vi "GIS Head Poll Process.vi"(7 "HeadNo":string, 8 "error in (no error)":errorcluster, 9 "notifierSync":refnum<notifier>, 10 "TopLevel":refnum<class "TopLevel.lvclass">, 11 "GIS Printer in":refnum<class "GIS Printer.lvclass">) -> (0 "error out":errorcluster, 3 "GIS Printer out":refnum<class "GIS Printer.lvclass">)   [LabVIEW 2022 SP3, in "GIS Printer.lvclass"]
uses:
  GIS Printer.lvclass
  TopLevel/TopLevel.lvclass
  Typedefs/PollCommandData-Cluster.ctl
  Typedefs/GIS_PollTimers--cluster.ctl
panel:
  in  "C1":bool
  in  "A1":bool
  in  "C2":bool
  in  "A2":bool
  in  "C3":bool
  in  "A3":bool
  in  "C4":bool
  in  "A4":bool
  in  "C33":bool
  in  "I33 3":bool
  in  "I33 2":bool
  in  "I33 1":bool
  in  "A33":bool
  in  "C22":bool
  in  "A22":bool
  in  "C11":bool
  in  "A11":bool
  in  "OK":bool
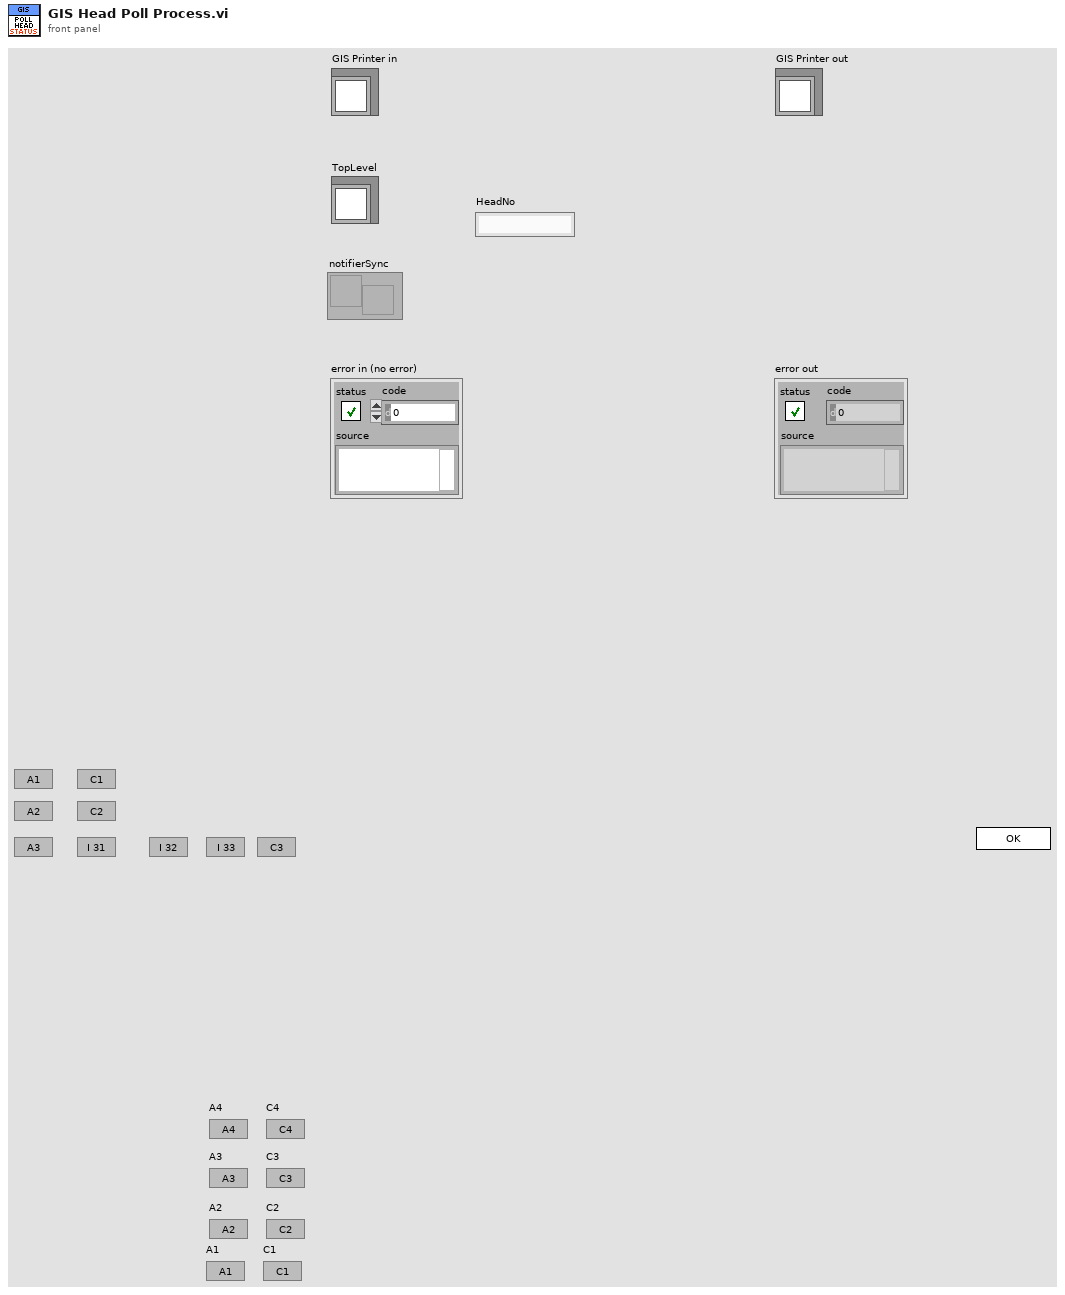
[diagram p1: front panel]
types:
  T1 = typedef "PollCommandData-Cluster.ctl" = cluster{"Command":string, "ID":i32, "Complete":bool}
  T2 = cluster{"String":string, "PrinterPollResponse":refnum<user-event>, "Open":bool, "TCP":refnum<k5>, "PollTrk":cluster{"CurrentCmdIndex":i32, "TotalCommands":i32}, "PollCommands":string[]}
  T3 = typedef "TD Dynamic CVT DVR--ref.ctl" = refnum<data-value>
  T4 = enum32{"Invalid", "Standard", "Closed", "Hidden", "Minimized", "Maximized"}
  T5 = enum32{"invalid app kind", "Development System", "Run Time System", "Student Edition", "Embedded LabVIEW", "Evaluation", "Custom"}
  T6 = typedef "GIS Printer.lvclass/PrinterConfiguration--Cluster.ctl" = cluster{"IPAddress":string, "Move Stage on RTP Command?":bool, "Stage Move Position":string, "PH1-Prime Path":path, "PH2-Prime Path":path, "PH3-Prime Path":path, "PH4-Prime Path":path, "PH5-Prime Path":path, "PH6-Prime Path":path, "PrintScriptsFolder":path, "PurgeScriptsFolder":path, "StageScriptsFolder":path, "PH1-HeatOn Path":path, "PH2-HeatOn Path":path, "PH3-HeatOn Path":path, "PH4-HeatOn Path":path, "PH5-HeatOn Path":path, "PH6-HeatOn Path":path, "PH1-HeatOff Path":path, "PH2-HeatOff Path":path, "PH3-HeatOff Path":path, "PH4-HeatOff Path":path, "PH5-HeatOff Path":path, "PH6-HeatOff Path":path}
  T7 = typedef "GIS_PollTimers--cluster.ctl" = cluster{"HeadStatus":dbl}
  T8 = cluster{"GIS Printer in":refnum<class "GIS Printer.lvclass">, "Core":cluster{"Current VI Reference":refnum<vi>, "Close Panel on Exit?":bool}, "PrinterConfiguration":T6, "TCP":refnum<k5>, "PollTimers":T7, "PollTracker":cluster{"HeadStatusPollStart":dbl, "Poll":bool}, "notifierSync":refnum<notifier>, "PollEnable":bool}
  T9 = cluster{"Current VI Reference":refnum<vi>, "Close Panel on Exit?":bool}
  T10 = typedef "TopLevel.lvclass/Digilens Config Cluster.ctl" = cluster{"Motion Controller":T11, "IO Config":T12, "PrinterConfiguration":T6, "DAQ Settings":T15}
  T11 = typedef "Motor Controller.lvclass/Motor Controller Config Data.ctl" = cluster{"Motor IP Addresss":string, "Current Position":i32, "Pulse_Per_mm":i32, "PrePrint":dbl[], "Load Position_mm":i32, "Laminate Position_mm":i32}
  T12 = typedef "IO.lvclass/IO Config Data.ctl" = cluster{"DAQDevices":T13[], "DI Channels":T14[], "DO Channels":T14[], "Material Names":string[], "AI Channels":T14[], "AO Channels":T14[]}
  T13 = typedef "IO.lvclass/DCON_DeviceConfig--Cluster.ctl" = cluster{"COM":string, "DeviceName":string, "BaudRate":u32, "Number of Channels":i32, "DeviceAddress":i32, "Enable":bool}
  T14 = typedef "IO.lvclass/Channel Data.ctl" = cluster{"Channel Name":string, "Device Name":string, "Channel No":string}
  T15 = typedef "DAQ.lvclass/TD DAQ Settings--cluster.ctl" = cluster{"Simulate DAQ":bool, "DI Settings":T16[], "AI Settings":T17[], "Relay IONames":string[], "AO IONames":string[], "AO NChan SingleTask":bool}
  T16 = typedef "DAQ.lvclass/TD DI Instrument Settings--cluster.ctl" = cluster{"Disable":bool, "DI TaskName":string, "DI RefreshIntv":i32}
  T17 = typedef "DAQ.lvclass/TD AI Instrument Settings--cluster.ctl" = cluster{"Disable":bool, "AI TaskName":string, "AI InstSettings":T18, "SimAI Ranges":T19}
  T18 = typedef "DAQ.lvclass/TD AI InstSettings--cluster.ctl" = cluster{"DaqRate":dbl, "NumSamples":i32}
  T19 = typedef "DAQ.lvclass/TD SimAI Ranges--cluster.ctl" = cluster{"lo":dbl, "hi":dbl}
  T20 = typedef "TopLevel.lvclass/UserEvents.ctl" = cluster{"API Incoming Event":refnum<user-event>, "API Executed Event":refnum<user-event>, "API Return Event":refnum<user-event>, "Exit Event":refnum<user-event>, "StatusChanged":refnum<user-event>, "DLP GUI Config Changed":refnum<user-event>, "AppEvent":refnum<user-event>, "Login Event":refnum<user-event>}
  T21 = typedef "GIS Printer.lvclass/UserEvents.ctl" = cluster{"API Incoming Event":refnum<user-event>, "API Executed Event":refnum<user-event>, "API Return Event":refnum<user-event>, "Status Changed Event":refnum<user-event>, "Abort":refnum<user-event>, "stop process":refnum<user-event>, "GISPollStatus":refnum<user-event>, "GISHeadStatus":refnum<user-event>, "Error Event":refnum<user-event>}
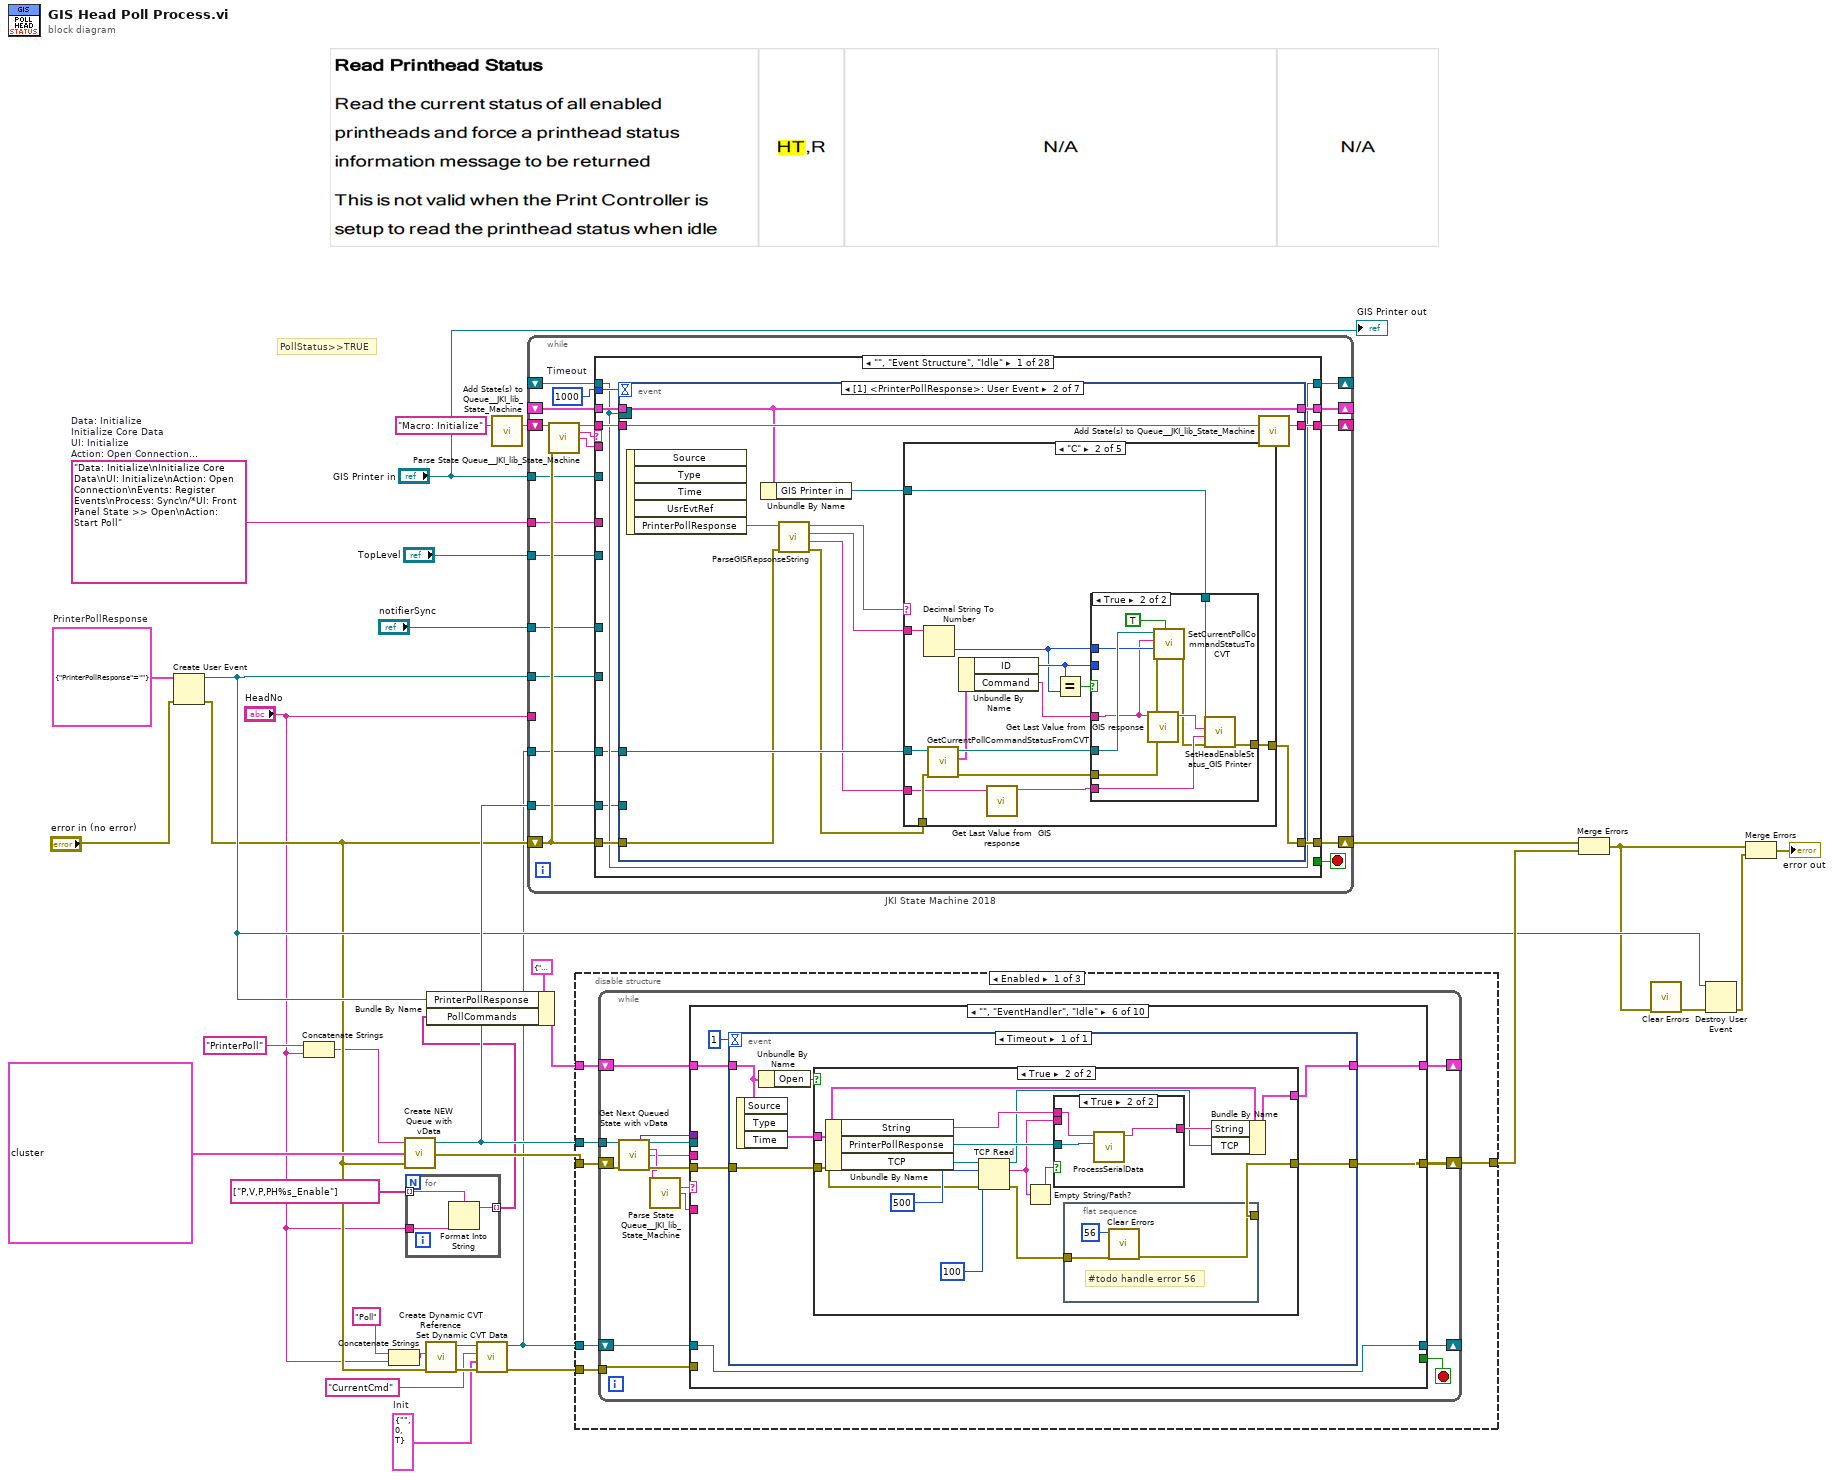
[diagram p0: block diagram]
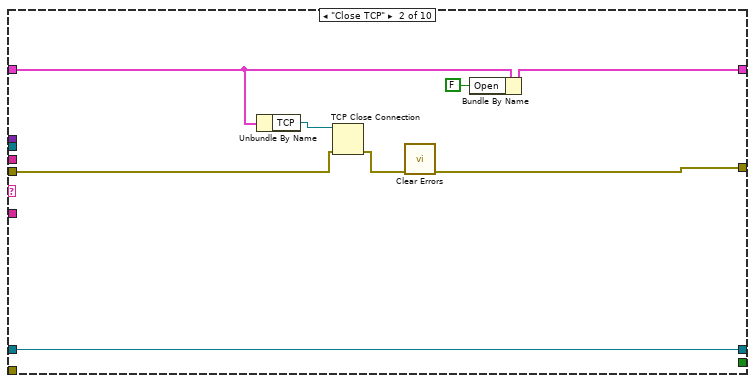
[diagram p3: hidden frame]
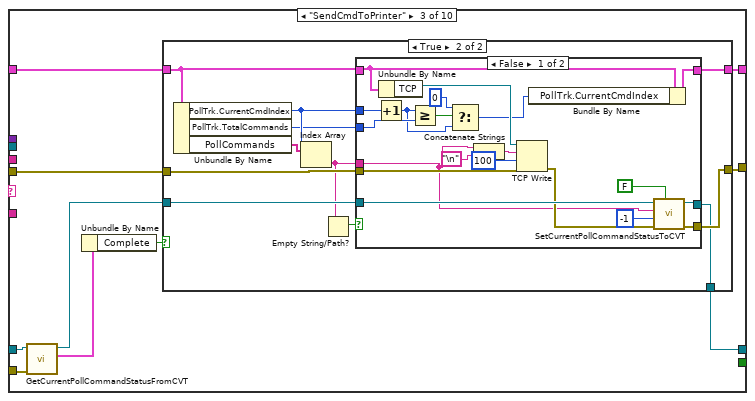
[diagram p4: hidden frame]
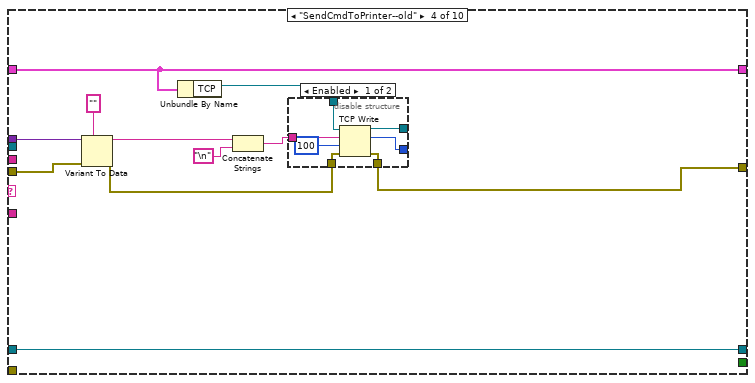
[diagram p7: hidden frame]
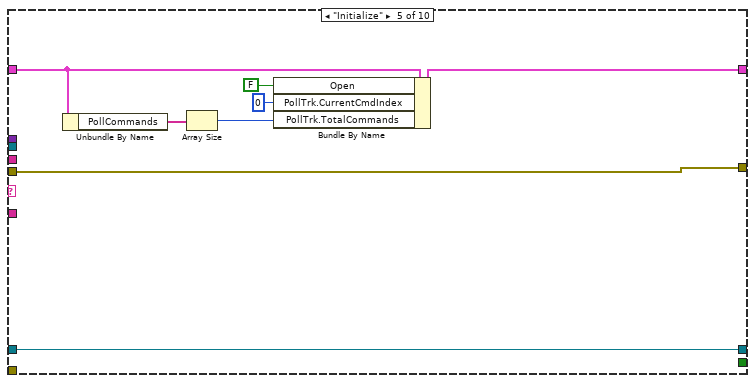
[diagram p9: hidden frame]
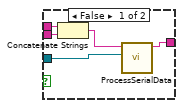
[diagram p11: hidden frame]
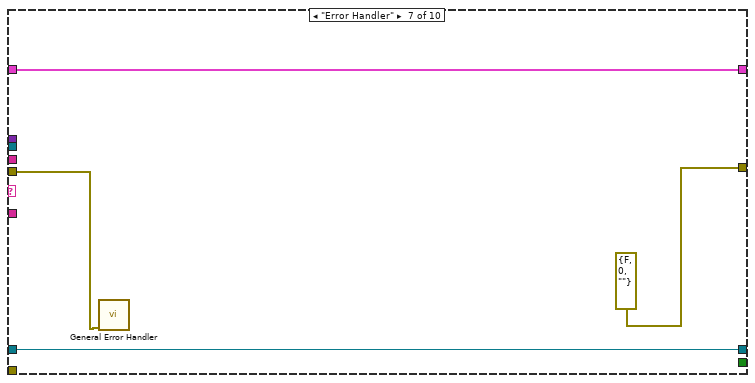
[diagram p12: hidden frame]
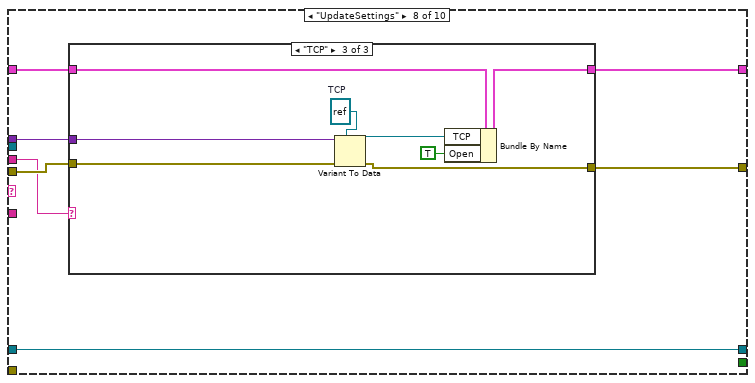
[diagram p13: hidden frame]
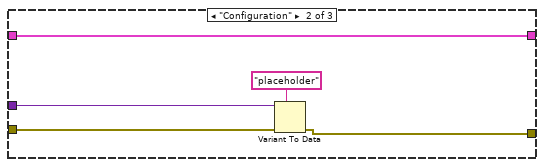
[diagram p15: hidden frame]
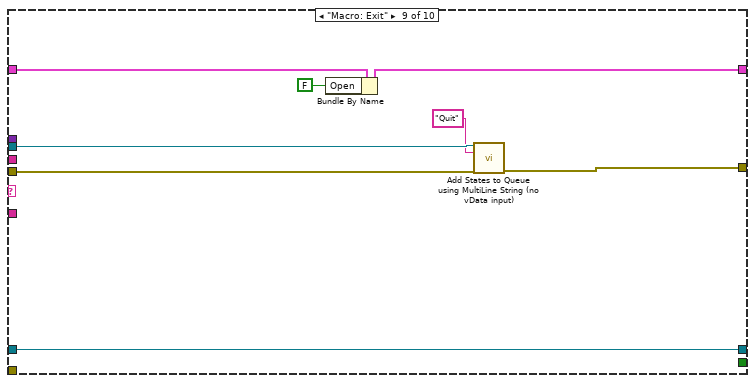
[diagram p16: hidden frame]
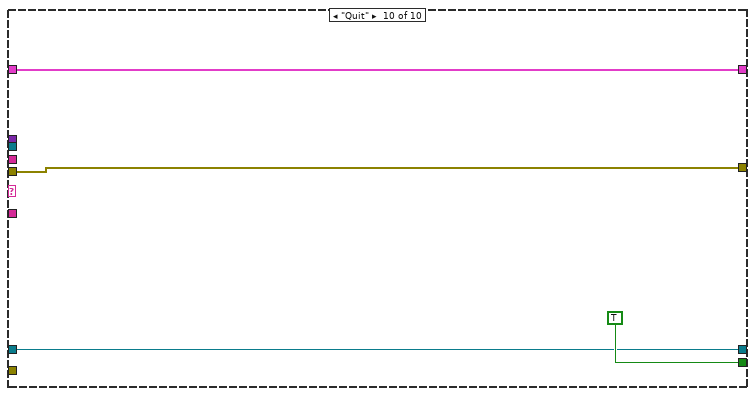
[diagram p17: hidden frame]
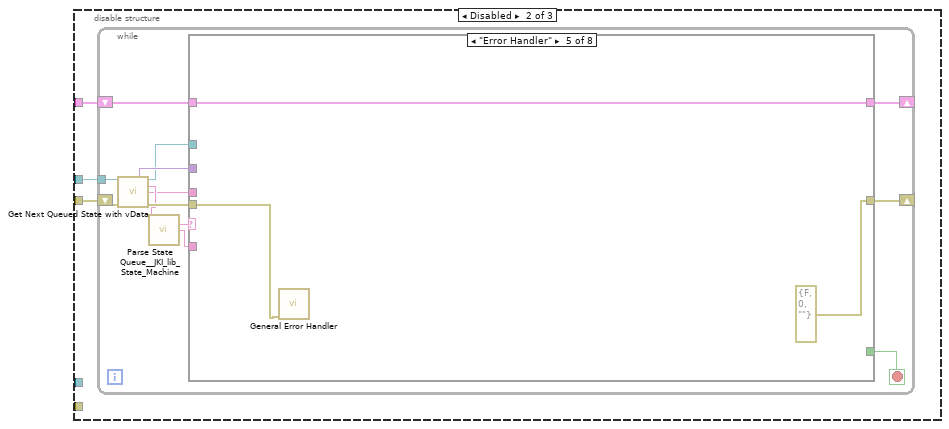
[diagram p18: hidden frame]
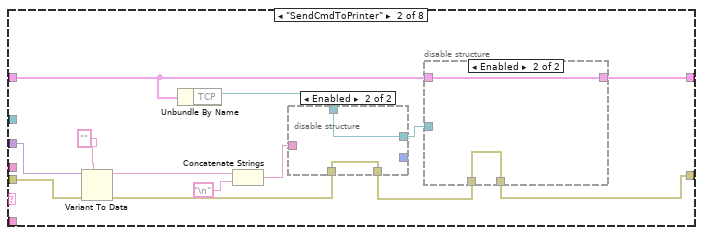
[diagram p20: hidden frame]
diagram:
  w7 = T1 {"Command"="", "ID"=0, "Complete"=TRUE}  # Init
  w14 = "Data: Initialize\nInitialize Core Data\nUI: Initialize\nAction: Open Connection\nEvents: Register Events\nProcess: Sync\n/*UI: Front Panel State >> Open\nAction: Start Poll"  # Data: Initialize Initialize Core Data UI: Initialize Action: Open Connection Events: Register Events Process: Sync /*UI: Front Panel State >> Open Action: Start Poll
  w25 = cluster{"PrinterPollResponse":string} {"PrinterPollResponse"=""}  # PrinterPollResponse
  # "PollStatus>>TRUE"
  n1 = Create User Event(user event datatype=w25, error in="error in (no error)") -> (user event=w22:refnum<user-event>, error out=w8:errorcluster)
  n2 = Concatenate Strings("PrinterPoll" ("Name (SMQ)"), "HeadNo") -> (w5:string)
  n3 = Concatenate Strings("Poll" ("DictName"), "HeadNo") -> (w4:string)
  n4 = call <vilib>:"Create NEW Queue with vData.vi"("error in (no error)"=w8, "Initial States"=cluster{"state":string, "vData":variant}[] [{"state"="Initialize", "vData"=variant}, {"state"="Idle", "vData"=variant}], "Name (SMQ)"=w5) -> ("error out"=w30:errorcluster, "queue out"=w26:refnum<queue>)  [unwired: 1 in]
  n5 = for {
    tunnel: string[] ["P,V,P,PH%s_Enable"] -> [w37] mode=indexing
    tunnel: "HeadNo" -> [w36]
    tunnel: [w35] -> w1 mode=indexing
    n6 = Format Into String(format string=w37, w36) -> (resulting string=w35:string)  [unwired: 2 in, 1 out]
  }
  n7 = call <vilib>:"Create Dynamic CVT Reference.vi"("error in (no error)"=w8, "DictName"=w4) -> ("error out"=w11:errorcluster, "dCVT DVR out"=w12:T3)  [unwired: 8 in]
  n8 = Bundle By Name(cluster=T2 {"String"="", "PrinterPollResponse"=refnum, "Open"=FALSE, "TCP"=refnum, "PollTrk"={"CurrentCmdIndex"=0, "TotalCommands"=0}, "PollCommands"=[]}, "PrinterPollResponse"=w22, "PollCommands"=w1) -> (w27:T2)
  n9 = call <vilib>:"Set Dynamic CVT Data.vi"("error in (no error)"=w11, "value"=w7, "DataName"="CurrentCmd", "dCVT DVR"=w12) -> ("error out"=w10:errorcluster, "dCVT DVR out"=w6:T3)  [unwired: 5 in, 1 out]
  n10 = call <vilib>:"Add State(s) to Queue__JKI_lib_State_Machine.vi"("State(s) in (\"\")"="Macro: Initialize") -> ("States Out"=w34:string)  [unwired: 14 in]
  n11 = while "JKI State Machine 2018" {
    shift-right: [w50] -> _
    shift-left: _ -> [w49]
    shift-right: [w53] -> w24
    shift-left: w8 -> [w47]
    shift-right: [w52] -> _
    shift-left: w34 -> [w54]
    tunnel: "GIS Printer in" -> [w46]
    tunnel: "TopLevel" -> [w45]
    tunnel: w26 -> [w44]
    tunnel: w22 -> [w43]
    shift-right: [w42] -> _
    shift-left: _ -> [w41]
    tunnel: "notifierSync" -> [w40]
    tunnel: w14 -> [w39]
    tunnel: w6 -> [w38]
    tunnel: "HeadNo" -> [_]
    stop <- w51 stop-if-true
    w48 = 1000  # Timeout
    n12 = call <vilib>:"Parse State Queue__JKI_lib_State_Machine.vi"("State Queue"=w54, "Error In (no error)"=w47) -> ("Remaining States"=w56:string, "Current State"=w57:string, "Arguments"=w55:string)  [unwired: 11 in]
    n13 = case shown="\"\", \"Event Structure\", \"Idle\"" w57 {
      selector: w57 -> [_ _ w182 _ _ _ _ _ _ _ _ _ _ _ _ _ _ _ _ _ _ _ _ _ _ _ _ _]
      tunnel: w56 -> [w67 w180 w186 w206 w213 w222 w227 w234 w248 w263 w270 w275 w280 w287 w299 w369 w375 w386 w391 w399 w407 w421 w435 w444 w459 w465 w477 w488]
      tunnel: w55 -> [_ _ _ _ _ _ _ _ _ _ _ _ _ w282 w293 _ _ _ _ _ _ _ _ _ _ _ w473 _]
      tunnel: w49 -> [w65 w177 w184 w199 w210 w220 w224 w232 w241 _ w265 w272 w278 w285 w295 w366 w372 w383 w388 w396 w402 w417 w431 w441 w454 w463 w475 w478]
      tunnel: [w64 w178 w188 w203 errorcluster {"status"=FALSE, "code"=0, "source"=""} ("error out") w215 w225 w230 w237 w249 w266 w273 w277 w283 w296 w367 w373 w384 w389 w393 w401 w419 w433 w442 w450 w461 w471 w481] -> w53
      tunnel: w47 -> [w63 w178 w187 w203 w209 w214 w225 w229 w243 w249 w267 w273 w277 w284 w297 w367 w373 w384 w389 w392 w400 w419 w433 w442 w446 w460 w470 w480]
      tunnel: [w66 w179 w185 w205 w212 w221 w226 w233 w247 w262 w269 w274 w279 w286 w298 w368 w374 w385 w390 w398 w406 w420 w434 w443 w458 w464 w476 w487] -> w52
      tunnel: [_ _ _ _ _ TRUE _ _ _ _ _ _ _ _ _ _ _ _ _ _ _ _ _ _ _ _ _ _] -> w51
      tunnel: [w62 w177 w184 w204 w210 w220 w224 w232 w242 w261 w265 w272 w278 w285 w295 w366 w372 w383 w388 w396 w402 w417 w431 w439 w454 w463 w468 w479] -> w50
      tunnel: w48 -> [w61 _ _ _ _ _ _ _ _ _ _ _ _ _ _ _ _ _ _ _ _ _ _ _ _ _ _ _]
      tunnel: w46 -> [_ _ _ _ _ _ _ _ _ w250 _ _ _ _ _ _ _ _ _ _ _ _ _ _ _ _ _ _]
      tunnel: w45 -> [_ _ _ _ _ _ _ _ _ w259 _ _ _ _ _ _ _ _ _ _ _ _ _ _ w448 _ _ _]
      tunnel: w44 -> [w58 _ _ _ _ w216 _ _ w239 _ _ _ _ _ _ _ _ _ _ w394 _ _ _ _ _ _ w472 w482]
      tunnel: w43 -> [_ _ _ _ _ _ _ _ _ _ _ _ _ _ _ _ _ _ _ _ _ _ _ _ w457 _ _ _]
      tunnel: [w60 w176 w181 w193 w207 w218 w223 w228 w235 w255 w264 w271 w276 w281 w292 w365 w371 w376 w387 w397 w405 w418 w432 w440 w456 w462 w469 w486] -> w42
      tunnel: w41 -> [w60 w176 w181 w193 w207 w218 w223 w228 w235 w255 w264 w271 w276 w281 w292 w365 w371 w376 w387 w397 w405 w418 w432 w440 _ w462 w469 w486]
      tunnel: w40 -> [_ _ _ _ _ _ _ _ _ w252 _ _ _ _ _ _ _ _ _ _ _ _ _ _ _ _ _ _]
      tunnel: w39 -> [_ _ _ _ _ _ _ _ _ _ _ _ _ _ _ _ w370 _ _ _ _ _ _ _ _ _ _ _]
      tunnel: w38 -> [w59 _ _ _ _ _ _ _ _ _ _ _ _ _ _ _ _ _ _ _ _ _ _ _ _ _ _ _]
      frame "", "Event Structure", "Idle" {
        n14 = event shown="[1] <PrinterPollResponse>: User Event" {
          selector: w60 -> [_ _ _ _ _ _ _]
          dyn-events: _ -> [_ _ _ _ _ _ _]
          timeout: w61 -> [_ _ _ _ _ _ _]
          tunnel: w67 -> [w75 w88 w143 w148 w152 w160 w175]
          tunnel: [w74 w87 w142 w147 w151 w159 w174] -> w66
          tunnel: w65 -> [w71 w84 w140 w145 w149 w155 w172]
          tunnel: [w73 w82 w141 w146 w150 w154 w173] -> w64
          tunnel: w63 -> [w73 w77 w141 w146 w150 w153 w173]
          tunnel: [w71 w84 w140 w145 w149 w156 w172] -> w62
          tunnel: w59 -> [_ w81 _ _ _ _ _]
          tunnel: w58 -> [_ _ _ _ _ _ _]
          event Timeout {
            n15 = event-data() -> ()  [unwired: 1 in, 1 out]
            n16 = Unbundle By Name(w71) -> ("PollTracker.Poll"=w70:bool, "PollEnable"=w68:bool)
            n17 = And(x=w70, y=w68) -> (x .and. y?=w69:bool)
            n18 = case shown="True" w69 {
              tunnel: [_ "Action: CheckPollTimers" ("State(s) in Front (\"\")")] -> w72
              frame False {
              }
              frame True {
              }
            }
            n19 = call <vilib>:"Add State(s) to Queue__JKI_lib_State_Machine.vi"("State(s) in Front (\"\")"=w72, "State(s) in (\"\")"=w75) -> ("States Out"=w74:string)  [unwired: 13 in]
          }
          event User Event {
            n20 = event-data() -> ("PrinterPollResponse"=w86:string)  [unwired: 1 in, 4 out]
            n21 = Unbundle By Name(w84) -> ("GIS Printer in"=w83:refnum<class "GIS Printer.lvclass">)
            n22 = call "ParseGISRepsonseString.vi"("error in (no error)"=w77, "Response In"=w86) -> ("error out"=w78:errorcluster, "Status"=w79:string, "ID"=w80:string, "Category"=w85:string)  [unwired: 6 in]
            n23 = case shown="\"C\"" w85 {
              tunnel: w79 -> [_ w91 w118 _ _]
              tunnel: w83 -> [_ w94 _ w137 _]
              tunnel: w78 -> [w89 w96 w124 w133 w138]
              tunnel: [w89 w97 w121 w134 w138] -> w82
              tunnel: w81 -> [_ w98 w125 _ _]
              tunnel: w80 -> [_ w92 w119 _ _]
              frame Default {
              }
              frame "C" {
                n24 = Decimal String To Number(string=w92) -> (number=w99:i32)  [unwired: 2 in, 1 out]
                n25 = call "GetCurrentPollCommandStatusFromCVT.vi"("error in (no error)"=w96, "Data Value Reference in"=w98) -> ("error out"=w102:errorcluster, "Command"=w95:T1, "Data Value Reference out"=w103:T3)  [unwired: 7 in]
                n26 = Unbundle By Name(w95) -> ("ID"=w100:i32, "Command"=w93:string)
                n27 = call "Get Last Value from  GIS response.vi"("Command"=w91) -> ("String"=w90:string)  [unwired: 10 in]
                n28 = Equal?(x=w100, y=w99) -> (x = y?=w101:bool)
                n29 = case shown="True" w101 {
                  tunnel: w103 -> [_ w114]
                  tunnel: w102 -> [w104 w113]
                  tunnel: [w104 w105] -> w97
                  tunnel: w100 -> [_ _]
                  tunnel: w99 -> [_ w111]
                  tunnel: w93 -> [_ w109]
                  tunnel: w94 -> [_ w110]
                  tunnel: w90 -> [_ w107]
                  frame False {
                    # "Ack is for a\ndifferent cmd,\nshould never\nhappen"
                  }
                  frame True {
                    n30 = call "Get Last Value from  GIS response.vi"("Command"=w109) -> ("String"=w108:string)  [unwired: 10 in]
                    n31 = call "SetCurrentPollCommandStatusToCVT.vi"("Complete"=TRUE, "error in (no error)"=w113, "Ack"=w111, "Command"=w109, "Data Value Reference in"=w114) -> ("error out"=w106:errorcluster)  [unwired: 5 in, 1 out]
                    n32 = call-dynamic "SetHeadEnableStatus_GIS Printer.vi"("error in (no error)"=w106, "Value"=w107, "Command"=w108, "GIS Printer In"=w110) -> ("error out"=w105:errorcluster)  [unwired: 6 in, 1 out]
                  }
                }
              }
              frame "A" {
                n33 = Decimal String To Number(string=w119) -> (number=w115:i32)  [unwired: 2 in, 1 out]
                n34 = call "GetCurrentPollCommandStatusFromCVT.vi"("error in (no error)"=w124, "Data Value Reference in"=w125) -> ("error out"=w122:errorcluster, "Command"=w120:T1, "Data Value Reference out"=w123:T3)  [unwired: 7 in]
                n35 = Unbundle By Name(w120) -> ("Command"=w116:string)
                n36 = Equal?(x=w116, y=w118) -> (x = y?=w117:bool)
                n37 = case shown="False" w117 {
                  tunnel: w123 -> [_ w132]
                  tunnel: w122 -> [w126 w131]
                  tunnel: [w126 w130] -> w121
                  tunnel: w120 -> [_ _]
                  tunnel: w116 -> [_ w128]
                  tunnel: w115 -> [_ w127]
                  frame False {
                    # "Ack is for a\ndifferent cmd,\nshould never\nhappen"
                  }
                  frame True {
                    n38 = call "SetCurrentPollCommandStatusToCVT.vi"("Complete"=FALSE, "error in (no error)"=w131, "Ack"=w127, "Command"=w128, "Data Value Reference in"=w132) -> ("error out"=w130:errorcluster)  [unwired: 5 in, 1 out]
                  }
                }
              }
              frame "E" {
                # "Should be replaced with actual error"
                n39 = call-dynamic "Generate Error Event.vi"("Error"=errorcluster {"status"=FALSE, "code"=0, "source"=""}, "GIS Printer in"=w137) -> ("error out"=w136:errorcluster)  [unwired: 8 in, 1 out]
                n40 = Merge Errors(w133, w136) -> (w134:errorcluster)
              }
              frame "I" {
              }
            }
            n41 = call <vilib>:"Add State(s) to Queue__JKI_lib_State_Machine.vi"("State(s) in (\"\")"=w88) -> ("States Out"=w87:string)  [unwired: 14 in]
          }
          event "OK": Value Change {
            # "Exit Button Value Change (pressed) Event\n(this executes Macro: Exit to terminate the VI)"
            n42 = event-data() -> ()  [unwired: 1 in, 1 out]
            n43 = call <vilib>:"Add State(s) to Queue__JKI_lib_State_Machine.vi"("State(s) in Front (\"\")"="Macro: Exit", "State(s) in (\"\")"=w143) -> ("States Out"=w142:string)  [unwired: 13 in]
          }
          event User Event {
            # "Exit Button Value Change (pressed) Event\n(this executes Macro: Exit to terminate the VI)"
            n44 = event-data() -> ()  [unwired: 1 in, 5 out]
            n45 = call <vilib>:"Add State(s) to Queue__JKI_lib_State_Machine.vi"("State(s) in Front (\"\")"="Macro: Exit", "State(s) in (\"\")"=w148) -> ("States Out"=w147:string)  [unwired: 13 in]
          }
          event User Event {
            # "#TODO API: Abort called in  other process. do something about it man!\njust do something...anything"
            # "Exit Button Value Change (pressed) Event\n(this executes Macro: Exit to terminate the VI)"
            n46 = event-data() -> ()  [unwired: 1 in, 5 out]
            n47 = call <vilib>:"Add State(s) to Queue__JKI_lib_State_Machine.vi"("State(s) in (\"\")"=w152) -> ("States Out"=w151:string)  [unwired: 14 in]
          }
          event User Event {
            n48 = event-data() -> ("Command"=w158:string, "Data"=w157:variant)  [unwired: 1 in, 4 out]
            n49 = case shown="\"StatusPoll\"" w158 {
              tunnel: w157 -> [_ w169]
              tunnel: w155 -> [w162 w167]
              tunnel: [w162 w166] -> w156
              tunnel: w153 -> [w161 w164]
              tunnel: [w161 w163] -> w154
              frame Default {
              }
              frame "StatusPoll" {
                n50 = Variant To Data(error in=w164, type=FALSE, Variant=w169) -> (data=w165:bool, error out=w163:errorcluster)
                n51 = Bundle By Name(cluster=w167, "PollEnable"=w165) -> (w166:T8)
              }
            }
            n52 = call <vilib>:"Add State(s) to Queue__JKI_lib_State_Machine.vi"("State(s) in (\"\")"=w160) -> ("States Out"=w159:string)  [unwired: 14 in]
          }
          event Panel Close? {
            # "Discard the event because we'll close the front panel ourselves in Macro: Exit"
            # "Close Panel button (pressed) Event\n(this executes Macro: Exit to terminate the VI)"
            n53 = event-data() -> ()  [unwired: 1 in, 1 out]
            n54 = event-data("Discard?"=TRUE) -> ()  [unwired: 1 in, 1 out]
            n55 = call <vilib>:"Add State(s) to Queue__JKI_lib_State_Machine.vi"("State(s) in Front (\"\")"="Macro: Exit", "State(s) in (\"\")"=w175) -> ("States Out"=w174:string)  [unwired: 13 in]
          }
        }
      }
      frame "---------- Core ----------" {
        # "Do not put any code in this frame.\n(it is a separator no-op)"
        n56 = call <vilib>:"Add State(s) to Queue__JKI_lib_State_Machine.vi"("State(s) in (\"\")"=w180) -> ("States Out"=w179:string)  [unwired: 14 in]
      }
      frame Default {
        w191 = 42 items=["No error", "Argument error", "Memory is full", "Out of zone", "End of file", "File already open", "Generic file I/O error", "File not found", "File permission error", "Disk is full", "Duplicate path", "Too many files open", "System feature not enabled", "Resource file not found", "Cannot add resource", "Resource not found", "Image not found", "Image memory error", "Pen does not exist", "Config type invalid", "Config token not found", "Config parse error", "Config memory error", "Bad external code format", "Bad external code offset", "External code not present", "Null window", "Destroy window error", "Null menu", "Print aborted", "Bad print record", "Print driver error", "Windows error during printing", "Memory error during printing", "Print dialog error", "Generic print error", "Invalid device refnum", "Device not found", "Device parameter error", "Device unit error", "Cannot open device", "Device call aborted", "Generic error", "Cancelled by user", "Object ID too low", "Object ID too high", "Object not in heap", "Unknown heap", "Unknown object (invalid DefProc)", "Unknown object (DefProc not in table)", "Message out of range", "Invalid (null) method", "Unknown message", "Manager call not supported", "Bad address", "Network operation in progress", "Network operation timed out", "Connection is busy", "Network attribute not supported", "Network error", "Address in use", "System out of memory", "Connection aborted", "Connection refused", "Not connected", "Already connected", "Connection closed", "Initialization error (interapplication manager)", "Bad occurrence", "Wait on unbound occurrence handler", "Occurrence queue overflow", "Datalog type conflict", "Unused", "Unrecognized type (interapplication manager)", "Memory corrupt", "Failed to make temporary DLL", "Old CIN version", "Drag socket not found", "Failed to load drop-object", "Failed to register OLE object", "Failed to release OLE object", "Format specifier type mismatch", "Unknown format specifier", "Too few format specifiers", "Too many format specifiers", "Scan failed", "Newer CIN version", "Error converting to variant", "Runtime menu error", "Password tampered", "Variant attribute not found", "Incompatible variant data type", "Event data is not available", "Event Store is not present", "Occurrence is not found", "Event Queue is not created", "Event info is not available", "Refnum passed is NULL", "Error retrieving Class GUID", "Error retrieving CoClass GUID", "Error retrieving TypeLib GUID.", "Bad built application magic bytes.", "Specific driver is different from the specific driver associated with the Logical Name.", "There is no session opened to the class driver.", "Max Error", "MAX - Error with config objects", "MAX - Error loading configuration", "MAX - Group not supported"]
        # "Current State"
        # "Do not delete, rename, or modify this frame.\n(this is used to capture unhandled states and typos)"
        # "Handle mistyped state name (developer tool)"
        n57 = Format Into String(format string="Software Exception: Unhandled State \"%s\"." ("message"), error in=w187, w182) -> (resulting string=w190:string, error out=w189:errorcluster)  [unwired: 1 in]
        n58 = call <vilib>:"Error Cluster From Error Code.vi"("show call chain? (False)"=TRUE, "error in (no error)"=w189, "error message (\"\")"=w190, "error code (0)"=w191) -> ("error out"=w188:errorcluster)  [unwired: 5 in]
        n59 = call <vilib>:"Add State(s) to Queue__JKI_lib_State_Machine.vi"("State(s) in (\"\")"=w186) -> ("States Out"=w185:string)  [unwired: 14 in]
      }
      frame "Initialize Core Data" {
        # "Do not delete, rename, or modify this frame.\n(this is used to determine panel behavior on exit)"
        # "originally closed?"
        # "exe?"
        # "If panel starts closed or is an EXE, then close it when we exit"
        n60 = property class="VI"() -> ("FP.State"=w196:T4)  [unwired: 2 in, 2 out]
        n61 = property class="App"() -> ("App.Kind"=w202:T5)  [unwired: 2 in, 2 out]
        n62 = control-ref of="Current VI Reference"() -> (w197:refnum<vi>)
        n63 = Equal?(x=w196, y=T4."Closed" ("Front Panel Window:State")) -> (x = y?=w194:bool)
        n64 = Equal?(x=w202, y=T5."Run Time System" ("Application:Kind")) -> (x = y?=w200:bool)
        n65 = Or(x=w194, y=w200) -> (x .or. y?=w198:bool)
        n66 = Bundle By Name(cluster=w199, "Core.Current VI Reference"=w197, "Core.Close Panel on Exit?"=w198) -> (w204:T8)
        n67 = call <vilib>:"Add State(s) to Queue__JKI_lib_State_Machine.vi"("State(s) in (\"\")"=w206) -> ("States Out"=w205:string)  [unwired: 14 in]
      }
      frame "Error Handler" {
        # "Unhandled Error -- Display it"
        # "Handle any errors here.\nYou can also output any states to clean-up after errors occur"
        # "Clear error"
        n68 = call <vilib>:"General Error Handler.vi"("error in (no error)"=w209) -> ()  [unwired: 10 in, 5 out]
        n69 = call <vilib>:"Add State(s) to Queue__JKI_lib_State_Machine.vi"("State(s) in Front (\"\")"="/* Post Error States", "State(s) in (\"\")"=w213) -> ("States Out"=w212:string)  [unwired: 13 in]
      }
      frame "Exit" {
        n70 = call <vilib>:"Add States to Queue using MultiLine String (no vData input).vi"("queue in"=w216, "states in"="Quit", "error in"=w214) -> ("error out"=w215:errorcluster)  [unwired: 10 in, 2 out]
        n71 = call <vilib>:"Add State(s) to Queue__JKI_lib_State_Machine.vi"("State(s) in (\"\")"=w222) -> ("States Out"=w221:string)  [unwired: 14 in]
      }
      frame "---------- Data ----------" {
        # "Do not put any code in this frame.\n(It is a separator no-op. You can make a copy of this frame to create a new Data frame)"
        n72 = call <vilib>:"Add State(s) to Queue__JKI_lib_State_Machine.vi"("State(s) in (\"\")"=w227) -> ("States Out"=w226:string)  [unwired: 14 in]
      }
      frame "Data: GIS Disconnect" {
        # "Do not put any code in this frame.\n(It is a separator no-op. You can make a copy of this frame to create a new Data frame)"
        n73 = Unbundle By Name(w232) -> ("TCP"=w231:refnum<k5>)
        n74 = TCP Close Connection(connection ID=w231, error in (no error)=w229) -> (error out=w230:errorcluster)  [unwired: 1 in, 1 out]
        n75 = call <vilib>:"Add State(s) to Queue__JKI_lib_State_Machine.vi"("State(s) in (\"\")"=w234) -> ("States Out"=w233:string)  [unwired: 14 in]
      }
      frame "Data: GIS Connect" {
        n76 = Unbundle By Name(w241) -> ("PrinterConfiguration.IPAddress"=w246:string)
        n77 = TCP Open Connection(address=w246, remote port or service name=u16 2000, timeout ms (60000)=1000, error in (no error)=w243) -> (connection ID=w236:refnum<k5>, error out=w238:errorcluster)  [unwired: 1 in]
        n78 = call <vilib>:"Add State to Queue with vData.vi"("queue in"=w239, "state in"="UpdateSettings>>TCP", "vData (\"\")"=w236, "error in"=w238) -> ("error out"=w237:errorcluster)  [unwired: 8 in, 3 out]
        n79 = Bundle By Name(cluster=w241, "TCP"=w236) -> (w242:T8)
        n80 = call <vilib>:"Add State(s) to Queue__JKI_lib_State_Machine.vi"("State(s) in (\"\")"=w248) -> ("States Out"=w247:string)  [unwired: 14 in]
      }
      frame "Data: Initialize" {
        w251 = TRUE  # PollEnable
        w253 = cluster{"HeadStatusPollStart":dbl, "Poll":bool} {"HeadStatusPollStart"=0.0, "Poll"=FALSE}  # PollTracker
        w254 = T7 {"HeadStatus"=2.0}  # PollTimers
        w256 = refnum<k5> refnum  # TCP
        w260 = T9 {"Current VI Reference"=refnum, "Close Panel on Exit?"=FALSE}  # Core
        # "#TODO get from config"
        n81 = property class="TopLevel.lvclass"(reference=w259) -> ("Methods:Accessors:Digilens Config"=w258:T10)  [unwired: 1 in, 2 out]
        n82 = Unbundle By Name(w258) -> ("PrinterConfiguration"=w257:T6)
        n83 = Bundle("GIS Printer in"=w250, "Core"=w260, "PrinterConfiguration"=w257, "TCP"=w256, "PollTimers"=w254, "PollTracker"=w253, "notifierSync"=w252, "PollEnable"=w251) -> (w261:T8)  [unwired: 1 in]
        n84 = call <vilib>:"Add State(s) to Queue__JKI_lib_State_Machine.vi"("State(s) in (\"\")"=w263) -> ("States Out"=w262:string)  [unwired: 14 in]
      }
      frame "Data: Cleanup" {
        # "Cleanup any data and references, here.\n(this is called automatically, by the Macro: Exit)"
        n85 = Unbundle By Name(w265) -> ("Core.Current VI Reference"=w268:refnum<vi>)
        n86 = Close Reference(reference=w268, error in (no error)=w267) -> (error out=w266:errorcluster)
        n87 = call <vilib>:"Add State(s) to Queue__JKI_lib_State_Machine.vi"("State(s) in (\"\")"=w270) -> ("States Out"=w269:string)  [unwired: 14 in]
      }
      frame "---------- UI ----------" {
        # "Do not put any code in this frame.\n(It is a separator no-op. You can make a copy of this frame to create a new UI frame)"
        n88 = call <vilib>:"Add State(s) to Queue__JKI_lib_State_Machine.vi"("State(s) in (\"\")"=w275) -> ("States Out"=w274:string)  [unwired: 14 in]
      }
      frame "UI: Initialize" {
        n89 = call <vilib>:"Add State(s) to Queue__JKI_lib_State_Machine.vi"("State(s) in (\"\")"=w280) -> ("States Out"=w279:string)  [unwired: 14 in]
      }
      frame "UI: Cursor Set" {
        # "Argument"
        # "Set and Unset Cursor Busy.\n(Usage: \"UI: Cursor Set >> Busy|Idle\")"
        n90 = case shown="\"Idle\", Default" w282 {
          tunnel: w284 -> [w289 w291]
          tunnel: [w288 w290] -> w283
          frame "Idle", Default {
            n91 = call <vilib>:"Unset Busy.vi"("error in (no error)"=w289) -> ("error out"=w288:errorcluster)  [unwired: 10 in]
          }
          frame "Busy" {
            n92 = call <vilib>:"Set Busy.vi"("error in (no error)"=w291) -> ("error out"=w290:errorcluster)  [unwired: 9 in, 1 out]
          }
        }
        n93 = call <vilib>:"Add State(s) to Queue__JKI_lib_State_Machine.vi"("State(s) in (\"\")"=w287) -> ("States Out"=w286:string)  [unwired: 14 in]
      }
      frame "UI: Front Panel State" {
        # "Argument"
        # "Set Front Panel Open or Closed\n(Usage: \"UI: Front Panel State >> Open|Close\")"
        n94 = Unbundle By Name(w295) -> ("Core.Current VI Reference"=w294:refnum<vi>)
        n95 = case shown="\"Minimize\", \"Minimized\"" w293 {
          tunnel: w297 -> [w305 w320 w331 w344 w357]
          tunnel: [w307 w321 w333 w346 w359] -> w296
          tunnel: w294 -> [w306 w318 w332 w345 w358]
          frame "Open", "Standard", Default {
            w300 = T4."Standard" ("State")
            n96 = property class="VI"(reference=w306, error in=w305) -> (reference out=w303:refnum<vi>, error out=w304:errorcluster, "FP.State"=w302:T4)
            n97 = Not Equal?(x=w302, y=w300) -> (x != y?=w301:bool)
            n98 = case shown="True" w301 {
              tunnel: [w311 w313] -> w307
              tunnel: w304 -> [w310 w313]
              tunnel: w303 -> [w309 _]
              tunnel: w300 -> [w308 _]
              frame True {
                n99 = invoke class="VI" method="FP.Open"(reference=w309, error in=w310, "Activate"=TRUE, "State"=w308) -> (error out=w311:errorcluster)  [unwired: 1 in, 4 out]
              }
              frame False {
              }
            }
          }
          frame "Close", "Closed" {
            n100 = property class="VI"(reference=w318, error in=w320) -> (reference out=w317:refnum<vi>, error out=w319:errorcluster, "FP.State"=w315:T4)
            n101 = Not Equal?(x=w315, y=T4."Closed" ("Front Panel Window:State")) -> (x != y?=w314:bool)
            n102 = case shown="True" w314 {
              tunnel: [w322 w325] -> w321
              tunnel: w319 -> [w322 w324]
              tunnel: w317 -> [_ w323]
              frame False {
              }
              frame True {
                n103 = invoke class="VI" method="FP.Close"(reference=w323, error in=w324) -> (error out=w325:errorcluster)  [unwired: 1 in, 2 out]
              }
            }
          }
          frame "Hidden", "Hide" {
            w326 = T4."Hidden" ("State")
            n104 = property class="VI"(reference=w332, error in=w331) -> (reference out=w329:refnum<vi>, error out=w330:errorcluster, "FP.State"=w328:T4)
            n105 = Not Equal?(x=w328, y=w326) -> (x != y?=w327:bool)
            n106 = case shown="True" w327 {
              tunnel: [w337 w338] -> w333
              tunnel: w330 -> [w336 w338]
              tunnel: w329 -> [w335 _]
              tunnel: w326 -> [w334 _]
              frame True {
                n107 = invoke class="VI" method="FP.Open"(reference=w335, error in=w336, "State"=w334) -> (error out=w337:errorcluster)  [unwired: 2 in, 4 out]
              }
              frame False {
              }
            }
          }
          frame "Minimize", "Minimized" {
            w339 = T4."Minimized" ("State")
            n108 = property class="VI"(reference=w345, error in=w344) -> (reference out=w342:refnum<vi>, error out=w343:errorcluster, "FP.State"=w341:T4)
            n109 = Not Equal?(x=w341, y=w339) -> (x != y?=w340:bool)
            n110 = case shown="True" w340 {
              tunnel: [w350 w351] -> w346
              tunnel: w343 -> [w349 w351]
              tunnel: w342 -> [w348 _]
              tunnel: w339 -> [w347 _]
              frame True {
                n111 = invoke class="VI" method="FP.Open"(reference=w348, error in=w349, "State"=w347) -> (error out=w350:errorcluster)  [unwired: 2 in, 4 out]
              }
              frame False {
              }
            }
          }
          frame "Maximize", "Maximized" {
            w352 = T4."Maximized" ("State")
            n112 = property class="VI"(reference=w358, error in=w357) -> (reference out=w355:refnum<vi>, error out=w356:errorcluster, "FP.State"=w354:T4)
            n113 = Not Equal?(x=w354, y=w352) -> (x != y?=w353:bool)
            n114 = case shown="True" w353 {
              tunnel: [w363 w364] -> w359
              tunnel: w356 -> [w362 w364]
              tunnel: w355 -> [w361 _]
              tunnel: w352 -> [w360 _]
              frame True {
                n115 = invoke class="VI" method="FP.Open"(reference=w361, error in=w362, "State"=w360) -> (error out=w363:errorcluster)  [unwired: 2 in, 4 out]
              }
              frame False {
              }
            }
          }
        }
        n116 = call <vilib>:"Add State(s) to Queue__JKI_lib_State_Machine.vi"("State(s) in (\"\")"=w299) -> ("States Out"=w298:string)  [unwired: 14 in]
      }
      frame "---------- Macro ----------" {
        # "Do not put any code in this frame.\n(It is a separator no-op. You can make a copy of this frame to create a new Macro frame)"
        n117 = call <vilib>:"Add State(s) to Queue__JKI_lib_State_Machine.vi"("State(s) in (\"\")"=w369) -> ("States Out"=w368:string)  [unwired: 14 in]
      }
      frame "Macro: Initialize" {
        n118 = call <vilib>:"Add State(s) to Queue__JKI_lib_State_Machine.vi"("State(s) in Front (\"\")"=w370, "State(s) in (\"\")"=w375) -> ("States Out"=w374:string)  [unwired: 13 in]
      }
      frame "Macro: Exit" {
        n119 = Unbundle By Name(w383) -> ("Core.Close Panel on Exit?"=w382:bool)
        n120 = Select(t="UI: Front Panel State >> Close", s=w382, f="") -> (s? t:f=w379:string)
        n121 = call <vilib>:"Add State(s) to Queue__JKI_lib_State_Machine.vi"("State(s) in (\"\")"=w379, "State(s) at Back (\"\")"="Data: Cleanup\nEvents: Unregister Events\nAction: Close Connection\nExit") -> ("States Out"=w377:string)  [unwired: 13 in]
        n122 = call <vilib>:"Add State(s) to Queue__JKI_lib_State_Machine.vi"("State(s) in Front (\"\")"=w377, "State(s) in (\"\")"=w386) -> ("States Out"=w385:string)  [unwired: 13 in]
      }
      frame "----------Action----------" {
        n123 = call <vilib>:"Add State(s) to Queue__JKI_lib_State_Machine.vi"("State(s) in (\"\")"=w391) -> ("States Out"=w390:string)  [unwired: 14 in]
      }
      frame "Action: Close Connection" {
        n124 = call <vilib>:"Add States to Queue using MultiLine String (no vData input).vi"("queue in"=w394, "states in"="Close TCP", "error in"=w392) -> ("error out"=w393:errorcluster)  [unwired: 10 in, 2 out]
        n125 = call <vilib>:"Add State(s) to Queue__JKI_lib_State_Machine.vi"("State(s) in (\"\")"=w399) -> ("States Out"=w398:string)  [unwired: 14 in]
      }
      frame "Process: Sync" {
        n126 = Unbundle By Name(w402) -> ("notifierSync"=w403:refnum<notifier>)
        n127 = Send Notification(notification=TRUE, notifier=w403, error in (no error)=w400) -> (error out=w401:errorcluster)  [unwired: 1 out]
        n128 = call <vilib>:"Add State(s) to Queue__JKI_lib_State_Machine.vi"("State(s) in (\"\")"=w407) -> ("States Out"=w406:string)  [unwired: 14 in]
      }
      frame "Action: CheckPollTimers" {
        n129 = Unbundle By Name(w417) -> ("PollTracker.HeadStatusPollStart"=w414:dbl)
        n130 = Unbundle By Name(w417) -> ("PollTimers.HeadStatus"=w412:dbl)
        n131 = Get Date/Time In Seconds() -> (seconds since 1Jan1904=w416:timestamp)
        n132 = To Double Precision Float(number=w416) -> (double precision float=w415:dbl)
        n133 = Subtract(x=w415, y=w414) -> (x-y=w413:dbl)
        n134 = Greater?(x=w413, y=w412) -> ()  [unwired: 1 out]
        n135 = Select(t="Action: Send GIS Command", s=TRUE, f="") -> (s? t:f=w409:string)
        n136 = call <vilib>:"Add State(s) to Queue__JKI_lib_State_Machine.vi"("State(s) in Front (\"\")"=w409, "State(s) in (\"\")"=w421) -> ("States Out"=w420:string)  [unwired: 13 in]
      }
      frame "Action: SendPollCommand" {
        # "#TODO delete later debug only"
        n137 = Unbundle By Name(w431) -> ("PollTracker.HeadStatusPollStart"=w428:dbl)
        n138 = Unbundle By Name(w431) -> ("PollTimers.HeadStatus"=w426:dbl)
        n139 = Get Date/Time In Seconds() -> (seconds since 1Jan1904=w430:timestamp)
        n140 = To Double Precision Float(number=w430) -> (double precision float=w429:dbl)
        n141 = Subtract(x=w429, y=w428) -> (x-y=w427:dbl)
        n142 = Greater?(x=w427, y=w426) -> (0:w422:bool)
        n143 = Select(t="Action: Send GIS Command", s=w422, f="") -> (s? t:f=w423:string)
        n144 = call <vilib>:"Add State(s) to Queue__JKI_lib_State_Machine.vi"("State(s) in Front (\"\")"=w423, "State(s) in (\"\")"=w435) -> ("States Out"=w434:string)  [unwired: 13 in]
      }
      frame "Action: Start Poll" {
        n145 = Get Date/Time In Seconds() -> (seconds since 1Jan1904=w437:timestamp)
        n146 = To Double Precision Float(number=w437) -> (double precision float=w436:dbl)
        n147 = Bundle By Name(cluster=w441, "PollTracker.Poll"=TRUE, "PollTracker.HeadStatusPollStart"=w436) -> (w439:T8)
        n148 = call <vilib>:"Add State(s) to Queue__JKI_lib_State_Machine.vi"("State(s) in (\"\")"=w444) -> ("States Out"=w443:string)  [unwired: 14 in]
      }
      frame "Events: Register Events" {
        n149 = call-dynamic "GetEvents_TopLevel.vi"("error in (no error)"=w446, "TopLevel in"=w448) -> ("error out"=w447:errorcluster, "UserEvents"=w449:T20)  [unwired: 7 in, 1 out]
        n150 = Unbundle By Name(w454) -> ("GIS Printer in"=w455:refnum<class "GIS Printer.lvclass">)
        n151 = Unbundle By Name(w449) -> ("AppEvent"=w445:refnum<user-event>)
        n152 = call-dynamic "GetEvents_GIS Printer.vi"("error in (no error)"=w447, "TopLevel in"=w455) -> ("error out"=w450:errorcluster, "UserEvents"=w453:T21)  [unwired: 7 in, 1 out]
        n153 = Unbundle By Name(w453) -> ("Abort"=w452:refnum<user-event>, "stop process"=w451:refnum<user-event>)
        n154 = register-events(w457, w452, w451, w445) -> (reference out=w456:refnum<event-registration>)  [unwired: 2 in, 1 out]
        n155 = call <vilib>:"Add State(s) to Queue__JKI_lib_State_Machine.vi"("State(s) in (\"\")"=w459) -> ("States Out"=w458:string)  [unwired: 14 in]
      }
      frame "Events: Unregister Events" {
        n156 = Unregister For Events(event registration refnum=w462, error in=w460) -> (error out=w461:errorcluster)
        n157 = call <vilib>:"Add State(s) to Queue__JKI_lib_State_Machine.vi"("State(s) in (\"\")"=w465) -> ("States Out"=w464:string)  [unwired: 14 in]
      }
      frame "Action: Send GIS Command" {
        n158 = Get Date/Time In Seconds() -> (seconds since 1Jan1904=w467:timestamp)
        n159 = To Double Precision Float(number=w467) -> (double precision float=w466:dbl)
        n160 = call <vilib>:"Add State to Queue with vData.vi"("queue in"=w472, "state in"="SendCmdToPrinter", "vData (\"\")"=w473, "error in"=w470) -> ("error out"=w471:errorcluster)  [unwired: 8 in, 3 out]
        n161 = Bundle By Name(cluster=w475, "PollTracker.HeadStatusPollStart"=w466) -> (w468:T8)
        n162 = call <vilib>:"Add State(s) to Queue__JKI_lib_State_Machine.vi"("State(s) in (\"\")"=w477) -> ("States Out"=w476:string)  [unwired: 14 in]
      }
      frame "Action: Open Connection" {
        n163 = disable-structure shown="Enabled" {
          disable-tunnel: w480 -> [w495 w496]
          disable-tunnel: w478 -> [w494 _]
          disable-tunnel: [w492 w496] -> w485
          disable-tunnel: [w491 refnum<k5> refnum ("connection ID")] -> w484
          frame Enabled {
            (unwired) "localhost" ("address")
            n164 = Unbundle By Name(w494) -> ("PrinterConfiguration.IPAddress"=w489:string)
            n165 = TCP Open Connection(address=w489, remote port or service name=u16 2000, timeout ms (60000)=1000, error in (no error)=w495) -> (connection ID=w491:refnum<k5>, error out=w492:errorcluster)  [unwired: 1 in]
          }
          frame Disabled {
          }
        }
        n166 = call <vilib>:"Add State to Queue with vData.vi"("queue in"=w482, "state in"="UpdateSettings>>TCP", "vData (\"\")"=w484, "error in"=w485) -> ("error out"=w481:errorcluster)  [unwired: 8 in, 3 out]
        n167 = Bundle By Name(cluster=w478, "TCP"=w484) -> (w479:T8)
        n168 = call <vilib>:"Add State(s) to Queue__JKI_lib_State_Machine.vi"("State(s) in (\"\")"=w488) -> ("States Out"=w487:string)  [unwired: 14 in]
      }
    }
  }
  n169 = disable-structure shown="Enabled" {
    disable-tunnel: w30 -> [w503 w684 w990]
    disable-tunnel: w27 -> [w502 w683 w989]
    disable-tunnel: w26 -> [w501 w682 w988]
    disable-tunnel: [w500 _ _] -> w23
    disable-tunnel: w6 -> [w499 _ _]
    disable-tunnel: w10 -> [w498 _ _]
    frame Enabled {
      n170 = while {
        tunnel: w501 -> [w512]
        shift-right: [w516] -> w500
        shift-left: w503 -> [w518]
        shift-right: [w513] -> _
        shift-left: w502 -> [w514]
        shift-right: [w504] -> _
        shift-left: w499 -> [w506]
        tunnel: w498 -> [w505]
        stop <- w519 stop-if-true
        n171 = call <vilib>:"Get Next Queued State with vData.vi"("queue in"=w512, "error in (no error)"=w518) -> ("vData out"=w515:variant, "queue out"=w511:refnum<queue>, "Next State"=w510:string, "queued msg"=w507:string, "error out"=w517:errorcluster)  [unwired: 7 in, 2 out]
        n172 = call <vilib>:"Parse State Queue__JKI_lib_State_Machine.vi"("State Queue"=w510) -> ("Current State"=w509:string, "Arguments"=w508:string)  [unwired: 12 in, 1 out]
        n173 = case shown="\"\", \"EventHandler\", \"Idle\"" w509 {
          tunnel: [_ _ _ _ _ _ _ _ _ TRUE] -> w519
          tunnel: w517 -> [w522 w527 w536 w588 w605 w610 w646 w653 w674 w680]
          tunnel: [w522 w524 w539 w579 w605 w609 errorcluster {"status"=FALSE, "code"=0, "source"=""} ("error out") w652 w673 w680] -> w516
          tunnel: w515 -> [_ _ _ w586 _ _ _ w654 _ _]
          tunnel: w514 -> [w521 w529 w538 w584 w599 w608 w645 w651 w677 w679]
          tunnel: [w521 w526 w540 w584 w604 w607 w645 w650 w672 w679] -> w513
          tunnel: w511 -> [_ _ _ _ _ _ _ _ w676 _]
          tunnel: w508 -> [_ _ _ _ _ _ _ _ _ _]
          tunnel: w507 -> [_ _ _ _ _ _ _ w649 _ _]
          tunnel: w506 -> [w520 w523 w534 w578 w600 w606 w644 w648 w670 w678]
          tunnel: w505 -> [_ _ w533 _ _ _ _ _ _ _]
          tunnel: [w520 w523 w535 w578 w600 w606 w644 w648 w670 w678] -> w504
          frame Default {
          }
          frame "Close TCP" {
            n174 = Unbundle By Name(w529) -> ("TCP"=w530:refnum<k5>)
            n175 = TCP Close Connection(connection ID=w530, error in (no error)=w527) -> (error out=w528:errorcluster)  [unwired: 1 in, 1 out]
            n176 = call <vilib>:"Clear Errors.vi"("error in (no error)"=w528) -> ("error out"=w524:errorcluster)  [unwired: 5 in, 1 out]
            n177 = Bundle By Name(cluster=w529, "Open"=FALSE) -> (w526:T2)
          }
          frame "SendCmdToPrinter" {
            n178 = call "GetCurrentPollCommandStatusFromCVT.vi"("error in (no error)"=w533, "Data Value Reference in"=w534) -> ("Command"=w531:T1, "Data Value Reference out"=w532:T3)  [unwired: 7 in, 1 out]
            n179 = Unbundle By Name(w531) -> ("Complete"=w537:bool)
            n180 = case shown="True" w537 {
              tunnel: w536 -> [w542 w554]
              tunnel: w538 -> [w543 w551]
              tunnel: [w543 w547] -> w540
              tunnel: [w542 w552] -> w539
              tunnel: w532 -> [w541 w553]
              tunnel: [w541 w546] -> w535
              frame False {
              }
              frame True {
                n181 = Unbundle By Name(w551) -> ("PollTrk.CurrentCmdIndex"=w549:i32, "PollTrk.TotalCommands"=w548:i32, "PollCommands"=w550:string[])
                n182 = Index Array(array=w550, index=w549) -> (element=w545:string)
                n183 = Empty String/Path?(string/path=w545) -> (empty?=w544:bool)
                n184 = case shown="False" w544 {
                  tunnel: w554 -> [w574 w575]
                  tunnel: w553 -> [w570 w577]
                  tunnel: [w566 w575] -> w552
                  tunnel: w551 -> [w565 w576]
                  tunnel: w549 -> [w564 _]
                  tunnel: w548 -> [w563 _]
                  tunnel: [w562 w576] -> w547
                  tunnel: [w556 w577] -> w546
                  tunnel: w545 -> [w555 _]
                  frame False {
                    n185 = Increment(x=w564) -> (x+1=w559:i32)
                    n186 = Unbundle By Name(w565) -> ("TCP"=w573:refnum<k5>)
                    n187 = Greater Or Equal?(x=w559, y=w563) -> (x >= y?=w560:bool)
                    n188 = Select(t=0, s=w560, f=w559) -> (s? t:f=w557:i32)
                    n189 = Concatenate Strings(w555, "\n") -> (w572:string)
                    n190 = TCP Write(connection ID=w573, data in=w572, error in (no error)=w574, 9:100 ("timeout ms (25000)")) -> (error out=w567:errorcluster)  [unwired: 2 out]
                    n191 = Bundle By Name(cluster=w565, "PollTrk.CurrentCmdIndex"=w557) -> (w562:T2)
                    n192 = call "SetCurrentPollCommandStatusToCVT.vi"("Complete"=FALSE, "error in (no error)"=w567, "Ack"=-1, "Command"=w555, "Data Value Reference in"=w570) -> ("error out"=w566:errorcluster, "Data Value Reference out"=w556:T3)  [unwired: 5 in]
                  }
                  frame True {
                  }
                }
              }
            }
          }
          frame "SendCmdToPrinter--old" {
            n193 = Variant To Data(error in=w588, type="", Variant=w586) -> (data=w583:string, error out=w585:errorcluster)
            n194 = Unbundle By Name(w584) -> ("TCP"=w582:refnum<k5>)
            n195 = Concatenate Strings(w583, "\n") -> (w581:string)
            n196 = disable-structure shown="Enabled" {
              disable-tunnel: w582 -> [w595 w597]
              disable-tunnel: [w594 w597] -> _
              disable-tunnel: w585 -> [w592 w596]
              disable-tunnel: w581 -> [w591 _]
              disable-tunnel: [w590 w596] -> w579
              disable-tunnel: [w589 _] -> _
              frame Enabled {
                n197 = TCP Write(connection ID=w595, data in=w591, error in (no error)=w592, 9:100 ("timeout ms (25000)")) -> (connection ID out=w594:refnum<k5>, bytes written=w589:i32, error out=w590:errorcluster)
              }
              frame Disabled {
              }
            }
          }
          frame "Initialize" {
            n198 = Unbundle By Name(w599) -> ("PollCommands"=w598:string[])
            n199 = Array Size(array=w598) -> (size(s)=w601:i32)
            n200 = Bundle By Name(cluster=w599, "Open"=FALSE, "PollTrk.CurrentCmdIndex"=0, "PollTrk.TotalCommands"=w601) -> (w604:T2)
          }
          frame "", "EventHandler", "Idle" {
            n201 = event shown="[0] Timeout" {
              selector: _ -> [_]
              dyn-events: _ -> [_]
              timeout: 1 -> [_]
              tunnel: w608 -> [w615]
              tunnel: w610 -> [w613]
              tunnel: [w612] -> w609
              tunnel: [w616] -> w607
              event Timeout {
                n202 = event-data() -> ()  [unwired: 1 in, 3 out]
                n203 = Unbundle By Name(w615) -> ("Open"=w614:bool)
                n204 = case shown="True" w614 {
                  tunnel: w615 -> [w618 w632]
                  tunnel: [w618 w630] -> w616
                  tunnel: w613 -> [w617 w620]
                  tunnel: [w617 w619] -> w612
                  frame False {
                  }
                  frame True {
                    n205 = Unbundle By Name(w632) -> ("String"=w631:string, "PrinterPollResponse"=w628:refnum<user-event>, "TCP"=w627:refnum<k5>)
                    n206 = TCP Read(connection ID=w627, bytes to read=500, error in (no error)=w620, 9:100 ("timeout ms (25000)")) -> (connection ID out=w621:refnum<k5>, data out=w626:string, error out=w622:errorcluster)  [unwired: 1 in]
                    n207 = Empty String/Path?(string/path=w626) -> (empty?=w625:bool)
                    n208 = case shown="True" w625 {
                      tunnel: w631 -> [w639 w642]
                      tunnel: [w638 w643] -> w629
                      tunnel: w628 -> [w637 w641]
                      tunnel: w626 -> [w636 _]
                      frame False {
                        n209 = Concatenate Strings(w639, w636) -> (w640:string)
                        n210 = call "ProcessSerialData.vi"("SerialResponseEvent"=w637, "String in"=w640) -> ("String out"=w638:string)  [unwired: 9 in]
                      }
                      frame True {
                        n211 = call "ProcessSerialData.vi"("SerialResponseEvent"=w641, "String in"=w642) -> ("String out"=w643:string)  [unwired: 9 in]
                      }
                    }
                    n212 = flat-sequence {
                      tunnel: w622 -> [w635]
                      tunnel: [w633] -> w619
                      frame #0 {
                        # "#todo handle error 56"
                        n213 = call <vilib>:"Clear Errors.vi"("error in (no error)"=w635, "specific error code to clear (0: all)"=56) -> ("error out"=w633:errorcluster)  [unwired: 4 in, 1 out]
                      }
                    }
                    n214 = Bundle By Name(cluster=w632, "String"=w629, "TCP"=w621) -> (w630:T2)
                  }
                }
              }
            }
          }
          frame "Error Handler" {
            n215 = call <vilib>:"General Error Handler.vi"("error in (no error)"=w646) -> ()  [unwired: 10 in, 5 out]
          }
          frame "UpdateSettings" {
            n216 = case shown="\"TCP\"" w649 {
              tunnel: w654 -> [_ w658 w666]
              tunnel: w653 -> [w656 w659 w667]
              tunnel: [w656 w660 w668] -> w652
              tunnel: w651 -> [w655 w661 w669]
              tunnel: [w655 w661 w664] -> w650
              frame "False", Default {
              }
              frame "Configuration" {
                n217 = Variant To Data(error in=w659, type="placeholder", Variant=w658) -> (error out=w660:errorcluster)  [unwired: 1 out]
              }
              frame "TCP" {
                w665 = refnum<k5> refnum  # TCP
                n218 = Variant To Data(error in=w667, type=w665, Variant=w666) -> (data=w663:refnum<k5>, error out=w668:errorcluster)
                n219 = Bundle By Name(cluster=w669, "TCP"=w663, "Open"=TRUE) -> (w664:T2)
              }
            }
          }
          frame "Macro: Exit" {
            n220 = Bundle By Name(cluster=w677, "Open"=FALSE) -> (w672:T2)
            n221 = call <vilib>:"Add States to Queue using MultiLine String (no vData input).vi"("queue in"=w676, "states in"="Quit", "error in"=w674) -> ("error out"=w673:errorcluster)  [unwired: 10 in, 2 out]
          }
          frame "Quit" {
          }
        }
      }
    }
    frame Disabled {
      n222 = while {
        tunnel: w682 -> [w690]
        shift-right: [w694] -> _
        shift-left: w684 -> [w696]
        shift-right: [w691] -> _
        shift-left: w683 -> [w692]
        stop <- w697 stop-if-true
        n223 = call <vilib>:"Get Next Queued State with vData.vi"("queue in"=w690, "error in (no error)"=w696) -> ("vData out"=w693:variant, "queue out"=w689:refnum<queue>, "Next State"=w688:string, "queued msg"=w685:string, "error out"=w695:errorcluster)  [unwired: 7 in, 2 out]
        n224 = call <vilib>:"Parse State Queue__JKI_lib_State_Machine.vi"("State Queue"=w688) -> ("Current State"=w687:string, "Arguments"=w686:string)  [unwired: 12 in, 1 out]
        n225 = case shown="\"Error Handler\"" w687 {
          tunnel: [_ _ _ _ _ _ _ TRUE] -> w697
          tunnel: w695 -> [w699 w712 w736 w740 w957 w963 w981 w986]
          tunnel: [w699 w702 w736 w739 errorcluster {"status"=FALSE, "code"=0, "source"=""} ("error out") w962 w980 w986] -> w694
          tunnel: w693 -> [_ w710 _ _ _ w964 _ _]
          tunnel: w692 -> [w698 w707 w735 w738 w956 w961 w984 w985]
          tunnel: [w698 w705 w734 w737 w956 w960 w984 w985] -> w691
          tunnel: w689 -> [_ _ _ _ _ _ w983 _]
          tunnel: w686 -> [_ _ _ _ _ _ _ _]
          tunnel: w685 -> [_ _ _ _ _ w959 _ _]
          frame Default {
          }
          frame "SendCmdToPrinter" {
            n226 = Variant To Data(error in=w712, type="", Variant=w710) -> (data=w709:string, error out=w708:errorcluster)
            n227 = Unbundle By Name(w707) -> ("TCP"=w706:refnum<k5>)
            n228 = Concatenate Strings(w709, "\n") -> (w701:string)
            n229 = disable-structure shown="Enabled" {
              disable-tunnel: w706 -> [w730 w732]
              disable-tunnel: [w729 w732] -> w704
              disable-tunnel: w708 -> [w727 w731]
              disable-tunnel: w701 -> [w726 _]
              disable-tunnel: [w725 w731] -> w703
              disable-tunnel: [w724 _] -> _
              frame Disabled {
                n230 = TCP Write(connection ID=w730, data in=w726, error in (no error)=w727, 9:100 ("timeout ms (25000)")) -> (connection ID out=w729:refnum<k5>, bytes written=w724:i32, error out=w725:errorcluster)
              }
              frame Enabled {
              }
            }
            n231 = disable-structure shown="Enabled" {
              disable-tunnel: w707 -> [w721 w723]
              disable-tunnel: [w720 w723] -> w705
              disable-tunnel: w704 -> [w717 _]
              disable-tunnel: w703 -> [w716 w722]
              disable-tunnel: [w715 w722] -> w702
              frame Disabled {
                n232 = TCP Read(connection ID=w717, bytes to read=100, error in (no error)=w716, 9:1000 ("timeout ms (25000)")) -> (connection ID out=w713:refnum<k5>, data out=w714:string, error out=w715:errorcluster)  [unwired: 1 in]
                n233 = Bundle By Name(cluster=w721, "TCP"=w713) -> (w720:T2)
                n234 = flat-sequence {
                  tunnel: w714 -> [_]
                  frame #0 {
                  }
                }
              }
              frame Enabled {
              }
            }
          }
          frame "Initialize" {
            n235 = Bundle By Name(cluster=w735, "Open"=FALSE) -> (w734:T2)
          }
          frame "", "EventHandler", "Idle" {
            n236 = event shown="[0] Timeout" {
              selector: _ -> [_ _ _ _ _ _ _ _ _ _]
              dyn-events: _ -> [_ _ _ _ _ _ _ _ _ _]
              timeout: 1 -> [_ _ _ _ _ _ _ _ _ _]
              tunnel: w738 -> [w743 w768 w789 w810 w831 w852 w873 w894 w915 w936]
              tunnel: w740 -> [w745 w770 w791 w812 w833 w854 w875 w896 w917 w938]
              tunnel: [w745 w770 w791 w812 w833 w854 w875 w896 w917 w938] -> w739
              tunnel: [w744 w769 w790 w811 w832 w853 w874 w895 w916 w937] -> w737
              event Timeout {
                n237 = event-data() -> ()  [unwired: 1 in, 3 out]
                n238 = Unbundle By Name(w743) -> ("Open"=w742:bool)
                n239 = case shown="True" w742 {
                  tunnel: w743 -> [w746 w758]
                  tunnel: [w746 w756] -> w744
                  frame False {
                  }
                  frame True {
                    n240 = Unbundle By Name(w758) -> ("String"=w757:string, "PrinterPollResponse"=w754:refnum<user-event>, "TCP"=w753:refnum<k5>)
                    n241 = TCP Read(connection ID=w753, bytes to read=500, 9:100 ("timeout ms (25000)")) -> (connection ID out=w747:refnum<k5>, data out=w752:string, error out=w748:errorcluster)  [unwired: 2 in]
                    n242 = Empty String/Path?(string/path=w752) -> (empty?=w751:bool)
                    n243 = case shown="False" w751 {
                      tunnel: w757 -> [w762 w765]
                      tunnel: [w761 w766] -> w755
                      tunnel: w754 -> [w760 w764]
                      tunnel: w752 -> [w759 _]
                      frame False {
                        n244 = Concatenate Strings(w762, w759) -> (w763:string)
                        n245 = call "ProcessSerialData.vi"("SerialResponseEvent"=w760, "String in"=w763) -> ("String out"=w761:string)  [unwired: 9 in]
                      }
                      frame True {
                        n246 = call "ProcessSerialData.vi"("SerialResponseEvent"=w764, "String in"=w765) -> ("String out"=w766:string)  [unwired: 9 in]
                      }
                    }
                    n247 = flat-sequence {
                      tunnel: w748 -> [_]
                      frame #0 {
                        # "#todo handle error 56"
                      }
                    }
                    n248 = Bundle By Name(cluster=w758, "String"=w755, "TCP"=w747) -> (w756:T2)
                  }
                }
              }
              event "A11": Value Change {
                n249 = event-data() -> ()  [unwired: 1 in, 6 out]
                n250 = Unbundle By Name(w768) -> ("Open"=w767:bool)
                n251 = case shown="True" w767 {
                  tunnel: w768 -> [w771 w779]
                  tunnel: [w771 w777] -> w769
                  frame False {
                  }
                  frame True {
                    w772 = "A,11,P,C,P,\"Print Manager,Print Line Manager,PMB-KM,PrintGoSource\",\"TTL\"\n"
                    n252 = Unbundle By Name(w779) -> ("String"=w778:string, "PrinterPollResponse"=w775:refnum<user-event>, "TCP"=w773:refnum<k5>)
                    n253 = Empty String/Path?(string/path=w772) -> (empty?=w774:bool)
                    n254 = case shown="False" w774 {
                      tunnel: w778 -> [w783 w786]
                      tunnel: [w782 w787] -> w776
                      tunnel: w775 -> [w781 w785]
                      tunnel: w772 -> [w780 _]
                      frame False {
                        n255 = Concatenate Strings(w783, w780) -> (w784:string)
                        n256 = call "ProcessSerialData.vi"("SerialResponseEvent"=w781, "String in"=w784) -> ("String out"=w782:string)  [unwired: 9 in]
                      }
                      frame True {
                        n257 = call "ProcessSerialData.vi"("SerialResponseEvent"=w785, "String in"=w786) -> ("String out"=w787:string)  [unwired: 9 in]
                      }
                    }
                    n258 = Bundle By Name(cluster=w779, "String"=w776, "TCP"=w773) -> (w777:T2)
                  }
                }
              }
              event "C11": Value Change {
                n259 = event-data() -> ()  [unwired: 1 in, 6 out]
                n260 = Unbundle By Name(w789) -> ("Open"=w788:bool)
                n261 = case shown="True" w788 {
                  tunnel: w789 -> [w792 w800]
                  tunnel: [w792 w798] -> w790
                  frame False {
                  }
                  frame True {
                    w793 = "C,11,0\n"
                    n262 = Unbundle By Name(w800) -> ("String"=w799:string, "PrinterPollResponse"=w796:refnum<user-event>, "TCP"=w794:refnum<k5>)
                    n263 = Empty String/Path?(string/path=w793) -> (empty?=w795:bool)
                    n264 = case shown="True" w795 {
                      tunnel: w799 -> [w804 w807]
                      tunnel: [w803 w808] -> w797
                      tunnel: w796 -> [w802 w806]
                      tunnel: w793 -> [w801 _]
                      frame False {
                        n265 = Concatenate Strings(w804, w801) -> (w805:string)
                        n266 = call "ProcessSerialData.vi"("SerialResponseEvent"=w802, "String in"=w805) -> ("String out"=w803:string)  [unwired: 9 in]
                      }
                      frame True {
                        n267 = call "ProcessSerialData.vi"("SerialResponseEvent"=w806, "String in"=w807) -> ("String out"=w808:string)  [unwired: 9 in]
                      }
                    }
                    n268 = Bundle By Name(cluster=w800, "String"=w797, "TCP"=w794) -> (w798:T2)
                  }
                }
              }
              event "A22": Value Change {
                n269 = event-data() -> ()  [unwired: 1 in, 6 out]
                n270 = Unbundle By Name(w810) -> ("Open"=w809:bool)
                n271 = case shown="True" w809 {
                  tunnel: w810 -> [w813 w821]
                  tunnel: [w813 w819] -> w811
                  frame False {
                  }
                  frame True {
                    w814 = "A,22,P,C,P,\"Print Manager,Print Line Manager,PMB-KM,EncoderSource\",\"RS422\"\n"
                    n272 = Unbundle By Name(w821) -> ("String"=w820:string, "PrinterPollResponse"=w817:refnum<user-event>, "TCP"=w815:refnum<k5>)
                    n273 = Empty String/Path?(string/path=w814) -> (empty?=w816:bool)
                    n274 = case shown="True" w816 {
                      tunnel: w820 -> [w825 w828]
                      tunnel: [w824 w829] -> w818
                      tunnel: w817 -> [w823 w827]
                      tunnel: w814 -> [w822 _]
                      frame False {
                        n275 = Concatenate Strings(w825, w822) -> (w826:string)
                        n276 = call "ProcessSerialData.vi"("SerialResponseEvent"=w823, "String in"=w826) -> ("String out"=w824:string)  [unwired: 9 in]
                      }
                      frame True {
                        n277 = call "ProcessSerialData.vi"("SerialResponseEvent"=w827, "String in"=w828) -> ("String out"=w829:string)  [unwired: 9 in]
                      }
                    }
                    n278 = Bundle By Name(cluster=w821, "String"=w818, "TCP"=w815) -> (w819:T2)
                  }
                }
              }
              event "C22": Value Change {
                n279 = event-data() -> ()  [unwired: 1 in, 6 out]
                n280 = Unbundle By Name(w831) -> ("Open"=w830:bool)
                n281 = case shown="True" w830 {
                  tunnel: w831 -> [w834 w842]
                  tunnel: [w834 w840] -> w832
                  frame False {
                  }
                  frame True {
                    w835 = "C,22,0\n"
                    n282 = Unbundle By Name(w842) -> ("String"=w841:string, "PrinterPollResponse"=w838:refnum<user-event>, "TCP"=w836:refnum<k5>)
                    n283 = Empty String/Path?(string/path=w835) -> (empty?=w837:bool)
                    n284 = case shown="True" w837 {
                      tunnel: w841 -> [w846 w849]
                      tunnel: [w845 w850] -> w839
                      tunnel: w838 -> [w844 w848]
                      tunnel: w835 -> [w843 _]
                      frame False {
                        n285 = Concatenate Strings(w846, w843) -> (w847:string)
                        n286 = call "ProcessSerialData.vi"("SerialResponseEvent"=w844, "String in"=w847) -> ("String out"=w845:string)  [unwired: 9 in]
                      }
                      frame True {
                        n287 = call "ProcessSerialData.vi"("SerialResponseEvent"=w848, "String in"=w849) -> ("String out"=w850:string)  [unwired: 9 in]
                      }
                    }
                    n288 = Bundle By Name(cluster=w842, "String"=w839, "TCP"=w836) -> (w840:T2)
                  }
                }
              }
              event "A33": Value Change {
                n289 = event-data() -> ()  [unwired: 1 in, 6 out]
                n290 = Unbundle By Name(w852) -> ("Open"=w851:bool)
                n291 = case shown="True" w851 {
                  tunnel: w852 -> [w855 w863]
                  tunnel: [w855 w861] -> w853
                  frame False {
                  }
                  frame True {
                    w856 = "A,33,P,P,1,C:\\Users\\labuser\\Desktop\\Scripts\\Patterns\\Print Weights\\PH1\\PW.bmp,5\n"
                    n292 = Unbundle By Name(w863) -> ("String"=w862:string, "PrinterPollResponse"=w859:refnum<user-event>, "TCP"=w857:refnum<k5>)
                    n293 = Empty String/Path?(string/path=w856) -> (empty?=w858:bool)
                    n294 = case shown="True" w858 {
                      tunnel: w862 -> [w867 w870]
                      tunnel: [w866 w871] -> w860
                      tunnel: w859 -> [w865 w869]
                      tunnel: w856 -> [w864 _]
                      frame False {
                        n295 = Concatenate Strings(w867, w864) -> (w868:string)
                        n296 = call "ProcessSerialData.vi"("SerialResponseEvent"=w865, "String in"=w868) -> ("String out"=w866:string)  [unwired: 9 in]
                      }
                      frame True {
                        n297 = call "ProcessSerialData.vi"("SerialResponseEvent"=w869, "String in"=w870) -> ("String out"=w871:string)  [unwired: 9 in]
                      }
                    }
                    n298 = Bundle By Name(cluster=w863, "String"=w860, "TCP"=w857) -> (w861:T2)
                  }
                }
              }
              event "I33 1": Value Change {
                n299 = event-data() -> ()  [unwired: 1 in, 6 out]
                n300 = Unbundle By Name(w873) -> ("Open"=w872:bool)
                n301 = case shown="True" w872 {
                  tunnel: w873 -> [w876 w884]
                  tunnel: [w876 w882] -> w874
                  frame False {
                  }
                  frame True {
                    w877 = "I,33,P\n"
                    n302 = Unbundle By Name(w884) -> ("String"=w883:string, "PrinterPollResponse"=w880:refnum<user-event>, "TCP"=w878:refnum<k5>)
                    n303 = Empty String/Path?(string/path=w877) -> (empty?=w879:bool)
                    n304 = case shown="True" w879 {
                      tunnel: w883 -> [w888 w891]
                      tunnel: [w887 w892] -> w881
                      tunnel: w880 -> [w886 w890]
                      tunnel: w877 -> [w885 _]
                      frame False {
                        n305 = Concatenate Strings(w888, w885) -> (w889:string)
                        n306 = call "ProcessSerialData.vi"("SerialResponseEvent"=w886, "String in"=w889) -> ("String out"=w887:string)  [unwired: 9 in]
                      }
                      frame True {
                        n307 = call "ProcessSerialData.vi"("SerialResponseEvent"=w890, "String in"=w891) -> ("String out"=w892:string)  [unwired: 9 in]
                      }
                    }
                    n308 = Bundle By Name(cluster=w884, "String"=w881, "TCP"=w878) -> (w882:T2)
                  }
                }
              }
              event "I33 2": Value Change {
                n309 = event-data() -> ()  [unwired: 1 in, 6 out]
                n310 = Unbundle By Name(w894) -> ("Open"=w893:bool)
                n311 = case shown="True" w893 {
                  tunnel: w894 -> [w897 w905]
                  tunnel: [w897 w903] -> w895
                  frame False {
                  }
                  frame True {
                    w898 = "I,33,RTP,1\n"
                    n312 = Unbundle By Name(w905) -> ("String"=w904:string, "PrinterPollResponse"=w901:refnum<user-event>, "TCP"=w899:refnum<k5>)
                    n313 = Empty String/Path?(string/path=w898) -> (empty?=w900:bool)
                    n314 = case shown="True" w900 {
                      tunnel: w904 -> [w909 w912]
                      tunnel: [w908 w913] -> w902
                      tunnel: w901 -> [w907 w911]
                      tunnel: w898 -> [w906 _]
                      frame False {
                        n315 = Concatenate Strings(w909, w906) -> (w910:string)
                        n316 = call "ProcessSerialData.vi"("SerialResponseEvent"=w907, "String in"=w910) -> ("String out"=w908:string)  [unwired: 9 in]
                      }
                      frame True {
                        n317 = call "ProcessSerialData.vi"("SerialResponseEvent"=w911, "String in"=w912) -> ("String out"=w913:string)  [unwired: 9 in]
                      }
                    }
                    n318 = Bundle By Name(cluster=w905, "String"=w902, "TCP"=w899) -> (w903:T2)
                  }
                }
              }
              event "I33 3": Value Change {
                n319 = event-data() -> ()  [unwired: 1 in, 6 out]
                n320 = Unbundle By Name(w915) -> ("Open"=w914:bool)
                n321 = case shown="True" w914 {
                  tunnel: w915 -> [w918 w926]
                  tunnel: [w918 w924] -> w916
                  frame False {
                  }
                  frame True {
                    w919 = "I,33,EP\n"
                    n322 = Unbundle By Name(w926) -> ("String"=w925:string, "PrinterPollResponse"=w922:refnum<user-event>, "TCP"=w920:refnum<k5>)
                    n323 = Empty String/Path?(string/path=w919) -> (empty?=w921:bool)
                    n324 = case shown="True" w921 {
                      tunnel: w925 -> [w930 w933]
                      tunnel: [w929 w934] -> w923
                      tunnel: w922 -> [w928 w932]
                      tunnel: w919 -> [w927 _]
                      frame False {
                        n325 = Concatenate Strings(w930, w927) -> (w931:string)
                        n326 = call "ProcessSerialData.vi"("SerialResponseEvent"=w928, "String in"=w931) -> ("String out"=w929:string)  [unwired: 9 in]
                      }
                      frame True {
                        n327 = call "ProcessSerialData.vi"("SerialResponseEvent"=w932, "String in"=w933) -> ("String out"=w934:string)  [unwired: 9 in]
                      }
                    }
                    n328 = Bundle By Name(cluster=w926, "String"=w923, "TCP"=w920) -> (w924:T2)
                  }
                }
              }
              event "C33": Value Change {
                n329 = event-data() -> ()  [unwired: 1 in, 6 out]
                n330 = Unbundle By Name(w936) -> ("Open"=w935:bool)
                n331 = case shown="True" w935 {
                  tunnel: w936 -> [w939 w947]
                  tunnel: [w939 w945] -> w937
                  frame False {
                  }
                  frame True {
                    w940 = "C,33,0\n"
                    n332 = Unbundle By Name(w947) -> ("String"=w946:string, "PrinterPollResponse"=w943:refnum<user-event>, "TCP"=w941:refnum<k5>)
                    n333 = Empty String/Path?(string/path=w940) -> (empty?=w942:bool)
                    n334 = case shown="True" w942 {
                      tunnel: w946 -> [w951 w954]
                      tunnel: [w950 w955] -> w944
                      tunnel: w943 -> [w949 w953]
                      tunnel: w940 -> [w948 _]
                      frame False {
                        n335 = Concatenate Strings(w951, w948) -> (w952:string)
                        n336 = call "ProcessSerialData.vi"("SerialResponseEvent"=w949, "String in"=w952) -> ("String out"=w950:string)  [unwired: 9 in]
                      }
                      frame True {
                        n337 = call "ProcessSerialData.vi"("SerialResponseEvent"=w953, "String in"=w954) -> ("String out"=w955:string)  [unwired: 9 in]
                      }
                    }
                    n338 = Bundle By Name(cluster=w947, "String"=w944, "TCP"=w941) -> (w945:T2)
                  }
                }
              }
            }
          }
          frame "Error Handler" {
            n339 = call <vilib>:"General Error Handler.vi"("error in (no error)"=w957) -> ()  [unwired: 10 in, 5 out]
          }
          frame "UpdateSettings" {
            n340 = case shown="\"TCP\"" w959 {
              tunnel: w964 -> [_ w968 w976]
              tunnel: w963 -> [w966 w969 w977]
              tunnel: [w966 w970 w978] -> w962
              tunnel: w961 -> [w965 w971 w979]
              tunnel: [w965 w971 w974] -> w960
              frame "False", Default {
              }
              frame "Configuration" {
                n341 = Variant To Data(error in=w969, type="placeholder", Variant=w968) -> (error out=w970:errorcluster)  [unwired: 1 out]
              }
              frame "TCP" {
                w975 = refnum<k5> refnum  # TCP
                n342 = Variant To Data(error in=w977, type=w975, Variant=w976) -> (data=w973:refnum<k5>, error out=w978:errorcluster)
                n343 = Bundle By Name(cluster=w979, "TCP"=w973, "Open"=TRUE) -> (w974:T2)
              }
            }
          }
          frame "Macro: Exit" {
            n344 = call <vilib>:"Add States to Queue using MultiLine String (no vData input).vi"("queue in"=w983, "states in"="Quit", "error in"=w981) -> ("error out"=w980:errorcluster)  [unwired: 10 in, 2 out]
          }
          frame "Quit" {
          }
        }
      }
    }
    frame Disabled {
      n345 = while {
        tunnel: w988 -> [w996]
        shift-right: [w1000] -> _
        shift-left: w990 -> [w1002]
        shift-right: [w997] -> _
        shift-left: w989 -> [w998]
        stop <- w1003 stop-if-true
        n346 = call <vilib>:"Get Next Queued State with vData.vi"("queue in"=w996, "error in (no error)"=w1002) -> ("vData out"=w999:variant, "queue out"=w995:refnum<queue>, "Next State"=w994:string, "queued msg"=w991:string, "error out"=w1001:errorcluster)  [unwired: 7 in, 2 out]
        n347 = call <vilib>:"Parse State Queue__JKI_lib_State_Machine.vi"("State Queue"=w994) -> ("Current State"=w993:string, "Arguments"=w992:string)  [unwired: 12 in, 1 out]
        n348 = case shown="\"\", \"EventHandler\", \"Idle\"" w993 {
          tunnel: [_ _ _ _ _ _ TRUE] -> w1003
          tunnel: w1001 -> [w1005 w1009 w1013 w1179 w1185 w1203 w1208]
          tunnel: [w1005 w1009 w1012 errorcluster {"status"=FALSE, "code"=0, "source"=""} ("error out") w1184 w1202 w1208] -> w1000
          tunnel: w999 -> [_ _ _ _ w1186 _ _]
          tunnel: w998 -> [w1004 w1008 w1011 w1178 w1183 w1206 w1207]
          tunnel: [w1004 w1007 w1010 w1178 w1182 w1206 w1207] -> w997
          tunnel: w995 -> [_ _ _ _ _ w1205 _]
          tunnel: w992 -> [_ _ _ _ _ _ _]
          tunnel: w991 -> [_ _ _ _ w1181 _ _]
          frame Default {
          }
          frame "Initialize" {
            n349 = Bundle By Name(cluster=w1008, "Open"=FALSE) -> (w1007:T2)
          }
          frame "", "EventHandler", "Idle" {
            n350 = event shown="[1] \"A4\": Value Change" {
              selector: _ -> [_ _ _ _ _ _ _ _ _]
              dyn-events: _ -> [_ _ _ _ _ _ _ _ _]
              timeout: 1 -> [_ _ _ _ _ _ _ _ _]
              tunnel: w1011 -> [w1016 w1035 w1053 w1071 w1089 w1107 w1125 w1143 w1161]
              tunnel: w1013 -> [w1018 w1037 w1055 w1073 w1091 w1109 w1127 w1145 w1163]
              tunnel: [w1018 w1037 w1055 w1073 w1091 w1109 w1127 w1145 w1163] -> w1012
              tunnel: [w1017 w1036 w1054 w1072 w1090 w1108 w1126 w1144 w1162] -> w1010
              event Timeout {
                n351 = event-data() -> ()  [unwired: 1 in, 3 out]
                n352 = Unbundle By Name(w1016) -> ("Open"=w1015:bool)
                n353 = case shown="True" w1015 {
                  tunnel: w1016 -> [w1019 w1027]
                  tunnel: [w1019 w1025] -> w1017
                  frame False {
                  }
                  frame True {
                    n354 = Unbundle By Name(w1027) -> ("String"=w1026:string, "PrinterPollResponse"=w1023:refnum<user-event>, "TCP"=w1022:refnum<k5>)
                    n355 = TCP Read(connection ID=w1022) -> (data out=w1021:string)  [unwired: 4 in, 2 out]
                    n356 = Empty String/Path?(string/path=w1021) -> (empty?=w1020:bool)
                    n357 = case shown="True" w1020 {
                      tunnel: w1026 -> [w1031 w1033]
                      tunnel: [w1030 w1033] -> w1024
                      tunnel: w1023 -> [w1029 _]
                      tunnel: w1021 -> [w1028 _]
                      frame False {
                        n358 = Concatenate Strings(w1031, w1028) -> (w1032:string)
                        n359 = call "ProcessSerialData.vi"("SerialResponseEvent"=w1029, "String in"=w1032) -> ("String out"=w1030:string)  [unwired: 9 in]
                      }
                      frame True {
                      }
                    }
                    n360 = Bundle By Name(cluster=w1027, "String"=w1024) -> (w1025:T2)
                  }
                }
              }
              event "A4": Value Change {
                n361 = event-data() -> ()  [unwired: 1 in, 6 out]
                n362 = Unbundle By Name(w1035) -> ("Open"=w1034:bool)
                n363 = case shown="True" w1034 {
                  tunnel: w1035 -> [w1038 w1045]
                  tunnel: [w1038 w1043] -> w1036
                  frame False {
                  }
                  frame True {
                    w1039 = "A,44,P,V,P,PH4_Temp_Read\n"
                    n364 = Unbundle By Name(w1045) -> ("String"=w1044:string, "PrinterPollResponse"=w1041:refnum<user-event>)
                    n365 = Empty String/Path?(string/path=w1039) -> (empty?=w1040:bool)
                    n366 = case shown="False" w1040 {
                      tunnel: w1044 -> [w1049 w1051]
                      tunnel: [w1048 w1051] -> w1042
                      tunnel: w1041 -> [w1047 _]
                      tunnel: w1039 -> [w1046 _]
                      frame False {
                        n367 = Concatenate Strings(w1049, w1046) -> (w1050:string)
                        n368 = call "ProcessSerialData.vi"("SerialResponseEvent"=w1047, "String in"=w1050) -> ("String out"=w1048:string)  [unwired: 9 in]
                      }
                      frame True {
                      }
                    }
                    n369 = Bundle By Name(cluster=w1045, "String"=w1042) -> (w1043:T2)
                  }
                }
              }
              event "C4": Value Change {
                n370 = event-data() -> ()  [unwired: 1 in, 6 out]
                n371 = Unbundle By Name(w1053) -> ("Open"=w1052:bool)
                n372 = case shown="True" w1052 {
                  tunnel: w1053 -> [w1056 w1063]
                  tunnel: [w1056 w1061] -> w1054
                  frame False {
                  }
                  frame True {
                    w1057 = "C,44,0,40\n"
                    n373 = Unbundle By Name(w1063) -> ("String"=w1062:string, "PrinterPollResponse"=w1059:refnum<user-event>)
                    n374 = Empty String/Path?(string/path=w1057) -> (empty?=w1058:bool)
                    n375 = case shown="False" w1058 {
                      tunnel: w1062 -> [w1067 w1069]
                      tunnel: [w1066 w1069] -> w1060
                      tunnel: w1059 -> [w1065 _]
                      tunnel: w1057 -> [w1064 _]
                      frame False {
                        n376 = Concatenate Strings(w1067, w1064) -> (w1068:string)
                        n377 = call "ProcessSerialData.vi"("SerialResponseEvent"=w1065, "String in"=w1068) -> ("String out"=w1066:string)  [unwired: 9 in]
                      }
                      frame True {
                      }
                    }
                    n378 = Bundle By Name(cluster=w1063, "String"=w1060) -> (w1061:T2)
                  }
                }
              }
              event "A3": Value Change {
                n379 = event-data() -> ()  [unwired: 1 in, 6 out]
                n380 = Unbundle By Name(w1071) -> ("Open"=w1070:bool)
                n381 = case shown="True" w1070 {
                  tunnel: w1071 -> [w1074 w1081]
                  tunnel: [w1074 w1079] -> w1072
                  frame False {
                  }
                  frame True {
                    w1075 = "A,33,P,V,P,PH3_Temp_Read\n"
                    n382 = Unbundle By Name(w1081) -> ("String"=w1080:string, "PrinterPollResponse"=w1077:refnum<user-event>)
                    n383 = Empty String/Path?(string/path=w1075) -> (empty?=w1076:bool)
                    n384 = case shown="False" w1076 {
                      tunnel: w1080 -> [w1085 w1087]
                      tunnel: [w1084 w1087] -> w1078
                      tunnel: w1077 -> [w1083 _]
                      tunnel: w1075 -> [w1082 _]
                      frame False {
                        n385 = Concatenate Strings(w1085, w1082) -> (w1086:string)
                        n386 = call "ProcessSerialData.vi"("SerialResponseEvent"=w1083, "String in"=w1086) -> ("String out"=w1084:string)  [unwired: 9 in]
                      }
                      frame True {
                      }
                    }
                    n387 = Bundle By Name(cluster=w1081, "String"=w1078) -> (w1079:T2)
                  }
                }
              }
              event "C3": Value Change {
                n388 = event-data() -> ()  [unwired: 1 in, 6 out]
                n389 = Unbundle By Name(w1089) -> ("Open"=w1088:bool)
                n390 = case shown="True" w1088 {
                  tunnel: w1089 -> [w1092 w1099]
                  tunnel: [w1092 w1097] -> w1090
                  frame False {
                  }
                  frame True {
                    w1093 = "C,33,0,30\n"
                    n391 = Unbundle By Name(w1099) -> ("String"=w1098:string, "PrinterPollResponse"=w1095:refnum<user-event>)
                    n392 = Empty String/Path?(string/path=w1093) -> (empty?=w1094:bool)
                    n393 = case shown="False" w1094 {
                      tunnel: w1098 -> [w1103 w1105]
                      tunnel: [w1102 w1105] -> w1096
                      tunnel: w1095 -> [w1101 _]
                      tunnel: w1093 -> [w1100 _]
                      frame False {
                        n394 = Concatenate Strings(w1103, w1100) -> (w1104:string)
                        n395 = call "ProcessSerialData.vi"("SerialResponseEvent"=w1101, "String in"=w1104) -> ("String out"=w1102:string)  [unwired: 9 in]
                      }
                      frame True {
                      }
                    }
                    n396 = Bundle By Name(cluster=w1099, "String"=w1096) -> (w1097:T2)
                  }
                }
              }
              event "A2": Value Change {
                n397 = event-data() -> ()  [unwired: 1 in, 6 out]
                n398 = Unbundle By Name(w1107) -> ("Open"=w1106:bool)
                n399 = case shown="True" w1106 {
                  tunnel: w1107 -> [w1110 w1117]
                  tunnel: [w1110 w1115] -> w1108
                  frame False {
                  }
                  frame True {
                    w1111 = "A,22,P,V,P,PH2_Temp_Read\n"
                    n400 = Unbundle By Name(w1117) -> ("String"=w1116:string, "PrinterPollResponse"=w1113:refnum<user-event>)
                    n401 = Empty String/Path?(string/path=w1111) -> (empty?=w1112:bool)
                    n402 = case shown="False" w1112 {
                      tunnel: w1116 -> [w1121 w1123]
                      tunnel: [w1120 w1123] -> w1114
                      tunnel: w1113 -> [w1119 _]
                      tunnel: w1111 -> [w1118 _]
                      frame False {
                        n403 = Concatenate Strings(w1121, w1118) -> (w1122:string)
                        n404 = call "ProcessSerialData.vi"("SerialResponseEvent"=w1119, "String in"=w1122) -> ("String out"=w1120:string)  [unwired: 9 in]
                      }
                      frame True {
                      }
                    }
                    n405 = Bundle By Name(cluster=w1117, "String"=w1114) -> (w1115:T2)
                  }
                }
              }
              event "C2": Value Change {
                n406 = event-data() -> ()  [unwired: 1 in, 6 out]
                n407 = Unbundle By Name(w1125) -> ("Open"=w1124:bool)
                n408 = case shown="True" w1124 {
                  tunnel: w1125 -> [w1128 w1135]
                  tunnel: [w1128 w1133] -> w1126
                  frame False {
                  }
                  frame True {
                    w1129 = "C,22,0,20\n"
                    n409 = Unbundle By Name(w1135) -> ("String"=w1134:string, "PrinterPollResponse"=w1131:refnum<user-event>)
                    n410 = Empty String/Path?(string/path=w1129) -> (empty?=w1130:bool)
                    n411 = case shown="False" w1130 {
                      tunnel: w1134 -> [w1139 w1141]
                      tunnel: [w1138 w1141] -> w1132
                      tunnel: w1131 -> [w1137 _]
                      tunnel: w1129 -> [w1136 _]
                      frame False {
                        n412 = Concatenate Strings(w1139, w1136) -> (w1140:string)
                        n413 = call "ProcessSerialData.vi"("SerialResponseEvent"=w1137, "String in"=w1140) -> ("String out"=w1138:string)  [unwired: 9 in]
                      }
                      frame True {
                      }
                    }
                    n414 = Bundle By Name(cluster=w1135, "String"=w1132) -> (w1133:T2)
                  }
                }
              }
              event "A1": Value Change {
                n415 = event-data() -> ()  [unwired: 1 in, 6 out]
                n416 = Unbundle By Name(w1143) -> ("Open"=w1142:bool)
                n417 = case shown="True" w1142 {
                  tunnel: w1143 -> [w1146 w1153]
                  tunnel: [w1146 w1151] -> w1144
                  frame False {
                  }
                  frame True {
                    w1147 = "A,11,P,V,P,PH1_Temp_Read\n"
                    n418 = Unbundle By Name(w1153) -> ("String"=w1152:string, "PrinterPollResponse"=w1149:refnum<user-event>)
                    n419 = Empty String/Path?(string/path=w1147) -> (empty?=w1148:bool)
                    n420 = case shown="False" w1148 {
                      tunnel: w1152 -> [w1157 w1159]
                      tunnel: [w1156 w1159] -> w1150
                      tunnel: w1149 -> [w1155 _]
                      tunnel: w1147 -> [w1154 _]
                      frame False {
                        n421 = Concatenate Strings(w1157, w1154) -> (w1158:string)
                        n422 = call "ProcessSerialData.vi"("SerialResponseEvent"=w1155, "String in"=w1158) -> ("String out"=w1156:string)  [unwired: 9 in]
                      }
                      frame True {
                      }
                    }
                    n423 = Bundle By Name(cluster=w1153, "String"=w1150) -> (w1151:T2)
                  }
                }
              }
              event "C1": Value Change {
                n424 = event-data() -> ()  [unwired: 1 in, 6 out]
                n425 = Unbundle By Name(w1161) -> ("Open"=w1160:bool)
                n426 = case shown="True" w1160 {
                  tunnel: w1161 -> [w1164 w1171]
                  tunnel: [w1164 w1169] -> w1162
                  frame False {
                  }
                  frame True {
                    w1165 = "C,11,0,10\n"
                    n427 = Unbundle By Name(w1171) -> ("String"=w1170:string, "PrinterPollResponse"=w1167:refnum<user-event>)
                    n428 = Empty String/Path?(string/path=w1165) -> (empty?=w1166:bool)
                    n429 = case shown="False" w1166 {
                      tunnel: w1170 -> [w1175 w1177]
                      tunnel: [w1174 w1177] -> w1168
                      tunnel: w1167 -> [w1173 _]
                      tunnel: w1165 -> [w1172 _]
                      frame False {
                        n430 = Concatenate Strings(w1175, w1172) -> (w1176:string)
                        n431 = call "ProcessSerialData.vi"("SerialResponseEvent"=w1173, "String in"=w1176) -> ("String out"=w1174:string)  [unwired: 9 in]
                      }
                      frame True {
                      }
                    }
                    n432 = Bundle By Name(cluster=w1171, "String"=w1168) -> (w1169:T2)
                  }
                }
              }
            }
          }
          frame "Error Handler" {
            n433 = call <vilib>:"General Error Handler.vi"("error in (no error)"=w1179) -> ()  [unwired: 10 in, 5 out]
          }
          frame "UpdateSettings" {
            n434 = case shown="\"TCP\"" w1181 {
              tunnel: w1186 -> [_ w1190 w1198]
              tunnel: w1185 -> [w1188 w1191 w1199]
              tunnel: [w1188 w1192 w1200] -> w1184
              tunnel: w1183 -> [w1187 w1193 w1201]
              tunnel: [w1187 w1193 w1196] -> w1182
              frame "False", Default {
              }
              frame "Configuration" {
                n435 = Variant To Data(error in=w1191, type="placeholder", Variant=w1190) -> (error out=w1192:errorcluster)  [unwired: 1 out]
              }
              frame "TCP" {
                w1197 = refnum<k5> refnum  # TCP
                n436 = Variant To Data(error in=w1199, type=w1197, Variant=w1198) -> (data=w1195:refnum<k5>, error out=w1200:errorcluster)
                n437 = Bundle By Name(cluster=w1201, "TCP"=w1195, "Open"=TRUE) -> (w1196:T2)
              }
            }
          }
          frame "Macro: Exit" {
            n438 = call <vilib>:"Add States to Queue using MultiLine String (no vData input).vi"("queue in"=w1205, "states in"="Quit", "error in"=w1203) -> ("error out"=w1202:errorcluster)  [unwired: 10 in, 2 out]
          }
          frame "Quit" {
          }
        }
      }
    }
  }
  n439 = Merge Errors(w24, w23) -> (w20:errorcluster)
  n440 = call <vilib>:"Clear Errors.vi"("error in (no error)"=w20) -> ("error out"=w21:errorcluster)  [unwired: 5 in, 1 out]
  n441 = Destroy User Event(user event=w22, error in=w21) -> (error out=w19:errorcluster)
  n442 = Merge Errors(w20, w19) -> (→"error out":errorcluster)
  "GIS Printer out" <- "GIS Printer in"
